vi "GUI_Beampointing2_Pico_HTU.vi"() -> ()   [LabVIEW 2020]
uses:
  Shared/GUI_Template/GUI_master/tcp_new_data_event.ctl
  Shared/GUI_Template/GUI_master/tcp new data cluster.ctl
  Ctrs/beam detection.ctl
  Ctrs/move_old.ctl
  Ctrs/stats.ctl
  General GUIs/Device GUIs/GUI_Cameras/Controls/Crosshair type def.ctl
  Ctrs/Motor Calibration.ctl
  <vilib>/Analysis/NI_AALBase.lvlib
panel:
  in  "size 2":cluster{"xhair size":dbl, "xhair size 2":dbl}={"xhair size"=20.0, "xhair size 2"=20.0} {"xhair size 2" min=0.0 max=0.0; "xhair size" min=0.0 max=0.0}
  in  "Time":timestamp[](array[timestamp])
  in  "Stats 2":T1
  in  "output cluster 2":T2
  in  "UDP error message":string
  in  "Save Stats":bool
  in  "output cluster":T6={"img to avg"=0, "beam detection para"={"Filter"=0, "Filter Para"={"X Size"=0, "Y Size"=0, "% Tolerance"=0}, "detection method"=0, "smal para"=[], "Remove small Objects"=FALSE, "Restrict to round Objects"=FALSE}, "move"={"Tolerance [%]"=0.1, "Stepsize"=0.0001, "Invert Axis"=TRUE, "Invert Direction X"=FALSE, "Invert Direction Y"=TRUE, "enable feedback"=FALSE, "Set Centriod Target"=FALSE, "my active motor"=""}, "GUIdevice 1"="", "GUIdevice 2"="", "ActiveMotor"=0, "stats path "=path ""} {"beam detection para"."smal para"."Measurement Parameter" items=["Center of Mass X", "Center of Mass Y", "First Pixel X", "First Pixel Y", "Bounding Rect Left", "Bounding Rect Top", "Bounding Rect Right", "Bounding Rect Bottom", "Max Feret Diameter Start X", "Max Feret Diameter Start Y", "Max Feret Diameter End X", "Max Feret Diameter End Y", "Max Horiz. Segment Length Left", "Max Horiz. Segment Length Right", "Max Horiz. Segment Length Row", "-", "Bounding Rect Width", "Bounding Rect Height", "Bounding Rect Diagonal", "Perimeter", "Convex Hull Perimeter", "Holes' Perimeter", "Max Feret Diameter", "Equivalent Ellipse Major Axis", "Equivalent Ellipse Minor Axis", "Equivalent Ellipse Minor Axis (Feret)", "Equivalent Rect Long Side", "Equivalent Rect Short Side", "Equivalent Rect Diagonal", "Equivalent Rect Short Side (Feret)", "Average Horiz. Segment Length", "Average Vert. Segment Length", "Hydraulic Radius", "Waddel Disk Diameter", "-", "Area", "Holes' Area", "Particle & Holes' Area", "Convex Hull Area", "Image Area", "-", "Number of Holes", "Number of Horiz. Segments", "Number of Vert. Segments", "-", "Orientation", "Max Feret Diameter Orientation", "-", "% Area/Image Area", "% Area/(Particle & Holes' Area)", "Ratio of Equivalent Ellipse Axes", "Ratio of Equivalent Rect Sides", "-", "Elongation Factor", "Compactness Factor", "Heywood Circularity Factor", "Type Factor", "-", "Sum X", "Sum Y", "Sum XX", "Sum XY", "Sum YY", "Sum XXX", "Sum XXY", "Sum XYY", "Sum YYY", "-", "Moment of Inertia XX", "Moment of Inertia XY", "Moment of Inertia YY", "Moment of Inertia XXX", "Moment of Inertia XXY", "Moment of Inertia XYY", "Moment of Inertia YYY", "Norm. Moment of Inertia XX", "Norm. Moment of Inertia XY", "Norm. Moment of Inertia YY", "Norm. Moment of Inertia XXX", "Norm. Moment of Inertia XXY", "Norm. Moment of Inertia XYY", "Norm. Moment of Inertia YYY", "Hu Moment 1", "Hu Moment 2", "Hu Moment 3", "Hu Moment 4", "Hu Moment 5", "Hu Moment 6", "Hu Moment 7"]; "beam detection para"."smal para"."Range Lower Value" format="%.2f"; "beam detection para"."smal para"."Range Upper Value" format="%.2f"; "beam detection para"."detection method" items=["clustering", "entropy", "metric", "moments", "inter-class variance"]; "beam detection para"."Filter" items=["No Filter", "Median Filter", "Low Pass Filter"]}
  in  "Trigger::1":bool
  in  "Triggerdelay::1":dbl=0.003 min=0.0 max=50000.0 format="%#_6f"
  in  "Exposure::1":dbl=0.095 min=0.0001 max=1.0 format="%#_6f"
  in  "ActiveMotorName::2":string
  in  "RelativeSettings.Axis 1.StepSize::2":dbl=50.0 caption="Axis 1 Stepsize" min=0.0 max=999999.0 format="%_4p"
  in  "RelativeSettings.Axis 3.StepSize::2":dbl=50.0 caption="Axis 2 StepSize" min=0.0 max=99999999.0 format="%_4p"
  in  "RelativeSettings.Axis 3.Position::2":dbl caption="Axis 2 Position" min=-9999990.0 max=999999.0 format="%_4p"
  in  "RelativeSettings.Axis 1.Position::2":dbl caption="Axis 1 Position" min=-999999.0 max=999999.0 format="%_4p"
  in  "RelativeMove.Axis 3.CW::2":bool caption="RelativeMove.Axis 2.CW::1"
  in  "RelativeMove.Axis 3.CCW::2":bool caption="RelativeMove.Axis. 2.CCW::1"
  in  "RelativeMove.Axis 1.CW::2":bool caption="RelativeMove.Axis 1.CW::1"
  in  "RelativeMove.Axis 1.CCW::2":bool caption="RelativeMove.Axis 1.CCW::1"
  out "Names":string[](array[string])=["PA2_Input1", "PA2_Input2", "L2_TelInpFar", "L1_TelInpNear", "L4_TREXPASS1", "L5_TREXPass2", "L6_TREXPass3", "L7_TREXPass4", "L8_M10Leak", "B1_TelInput", "B2_TelLens1"]
  in  "ActiveMotor":u16(ring)=7 items=["PA2_Input1", "PA2_Input2", "L2_TelInpFar", "L1_TelInpNear", "StretcherOut"]
  in  "Set Centriod Target":bool
  in  "size":dbl=10.299999999999997
  in  "Tab Control 2":enum32{"CCD Original ", "CCD Detected"}(tab)=enum."CCD Detected"
  out "image::1":T7(plugin-control) caption="StagingM1Far"
  out "Beam":T7(plugin-control)
  in  "Reset History":bool
  out "centriod X":dbl[](graph)=[249.59745762711864, 249.9873417721519, 249.85593220338984]
  out "centriod Y":dbl[](graph)=[256.39830508474574, 256.0126582278481, 257.0]
  out "Stats":cluster{timestamp[], dbl[]}[](graph)
  in  "Tab Control":enum32{"System", "Detection", "Feedback"}(tab)=enum."Feedback"
  in  "Save Stats":bool
  in  "update speed [ms]":i32=200
  in  "img to avg":i32=20
  in  "Save Config":bool
  in  "Load Config":bool
  in  "Cameras":u16(ring)=15 items=["10TW_Driver_Spot_Cam", "B1_TelInput", "B2_TelLens1", "B3_TelLens2", "B5_CompressorOut", "B6_SwitchYNear", "B9_OAPFront", "GIGEtest", "L1_TelInpNear", "L2_TelInpFar", "L3_TelescopeOut", "L4_TREXpass1", "L5_TREXPass2", "L6_TREXpass3", "L7_TREXPass4", "L8_M10Leak", "OAPtestCam", "PA2_Input1", "PA2_Input2", "PaperCam", "StagingAlignBeam1", "StagingAlignBeam2", "StagingCapAlignment", "StagingCapSpec", "StagingCapSpec1stOrder", "StagingChromaxGuppy", "StagingDiodeMonitor", "StagingFocusBeam1", "StagingFocusBeam2", "StagingGuppy", "StagingM1Far", "StagingM1Near", "StagingM3Far", "StagingM4", "StagingM5", "StagingMagnetCam1", "StagingMagnetCam2", "StagingMagnetCam3", "StagingManta2", "StagingModeImager2", "StagingModeTemp", "StagingOAP1Far", "StagingOAP1Near", "StagingOAP2Far", "StagingOAP2Near", "StagingPhasics", "StagingPhosphor", "StagingTapeCam", "StagingTapeMonitorCam", "StagingTopView", "TargetCam10Hz_Diode", "TargetCam1Hz_Pulsed", "TREXVarianCam0", "TREXVarianCam1", "TREXVarianCam2", "TREXVarianCam3", "TREX_CapSideView", "TREX_TA6", "TS-253a_in", "TS-CapSideview", "TS-CapSpec", "TS-ChromexCam", "TS-InputNearField", "TS-Mode1", "TS-OverlapCam", "TS-Periscope", "XUV_Cam1", "XUV_Cam2"]
  in  "calibrate":bool
  in  "stats path":path
  in  "beam detection para":T3={"Filter"=1, "Filter Para"={"X Size"=5, "Y Size"=5, "% Tolerance"=1}, "detection method"=4, "smal para"=[{"Measurement Parameter"=35, "Range Lower Value"=150.0, "Range Upper Value"=300.0, "Range"=FALSE, "Measurement Type"=FALSE}], "Remove small Objects"=TRUE, "Restrict to round Objects"=FALSE} {"smal para"."Measurement Parameter" items=["Center of Mass X", "Center of Mass Y", "First Pixel X", "First Pixel Y", "Bounding Rect Left", "Bounding Rect Top", "Bounding Rect Right", "Bounding Rect Bottom", "Max Feret Diameter Start X", "Max Feret Diameter Start Y", "Max Feret Diameter End X", "Max Feret Diameter End Y", "Max Horiz. Segment Length Left", "Max Horiz. Segment Length Right", "Max Horiz. Segment Length Row", "-", "Bounding Rect Width", "Bounding Rect Height", "Bounding Rect Diagonal", "Perimeter", "Convex Hull Perimeter", "Holes' Perimeter", "Max Feret Diameter", "Equivalent Ellipse Major Axis", "Equivalent Ellipse Minor Axis", "Equivalent Ellipse Minor Axis (Feret)", "Equivalent Rect Long Side", "Equivalent Rect Short Side", "Equivalent Rect Diagonal", "Equivalent Rect Short Side (Feret)", "Average Horiz. Segment Length", "Average Vert. Segment Length", "Hydraulic Radius", "Waddel Disk Diameter", "-", "Area", "Holes' Area", "Particle & Holes' Area", "Convex Hull Area", "Image Area", "-", "Number of Holes", "Number of Horiz. Segments", "Number of Vert. Segments", "-", "Orientation", "Max Feret Diameter Orientation", "-", "% Area/Image Area", "% Area/(Particle & Holes' Area)", "Ratio of Equivalent Ellipse Axes", "Ratio of Equivalent Rect Sides", "-", "Elongation Factor", "Compactness Factor", "Heywood Circularity Factor", "Type Factor", "-", "Sum X", "Sum Y", "Sum XX", "Sum XY", "Sum YY", "Sum XXX", "Sum XXY", "Sum XYY", "Sum YYY", "-", "Moment of Inertia XX", "Moment of Inertia XY", "Moment of Inertia YY", "Moment of Inertia XXX", "Moment of Inertia XXY", "Moment of Inertia XYY", "Moment of Inertia YYY", "Norm. Moment of Inertia XX", "Norm. Moment of Inertia XY", "Norm. Moment of Inertia YY", "Norm. Moment of Inertia XXX", "Norm. Moment of Inertia XXY", "Norm. Moment of Inertia XYY", "Norm. Moment of Inertia YYY", "Hu Moment 1", "Hu Moment 2", "Hu Moment 3", "Hu Moment 4", "Hu Moment 5", "Hu Moment 6", "Hu Moment 7"]; "smal para"."Range Lower Value" format="%.2f"; "smal para"."Range Upper Value" format="%.2f"; "detection method" items=["clustering", "entropy", "metric", "moments", "inter-class variance"]; "Filter" items=["No Filter", "Median Filter", "Low Pass Filter"]}
  in  "Move Properties":T5={"Tolerance [%]"=0.1, "Stepsize"=0.0001, "Invert Axis"=TRUE, "Invert Direction X"=FALSE, "Invert Direction Y"=TRUE, "enable feedback"=FALSE, "Set Centriod Target"=FALSE, "my active motor"=""} {"Stepsize" format="%#_6p"}
  out "Y Size":dbl=20.599999999999994
  out "X Size":dbl=15.599999999999994
  out "Particle Reports (Pixels)":T8(array[cluster])=[{"Area"=236.0, "Number of Holes"=0.0, "Bounding Rect"={"Left"=243.0, "Top"=247.0, "Right"=258.0, "Bottom"=268.0}, "Center of Mass"={"X"=249.85593220338984, "Y"=257.0}, "Orientation"=87.89795034558499, "Dimensions"={"Width"=15.0, "Height"=21.0}}] {"Orientation" format="%.2f"; "Dimensions"."Height" format="%.2f"; "Dimensions"."Width" format="%.2f"; "Center of Mass"."Y" format="%.2f"; "Center of Mass"."X" format="%.2f"; "Bounding Rect"."Bottom" format="%.2f"; "Bounding Rect"."Right" format="%.2f"; "Bounding Rect"."Top" format="%.2f"; "Bounding Rect"."Left" format="%.2f"; "Number of Holes" format="%.2f"; "Area" format="%.2f"}
  out "move required":bool=TRUE
  out "moving":bool
  out "Best Rectangle":T9(array[cluster])=[{"Left"=243.0, "Top"=247.0, "Right"=259.0, "Bottom"=267.0}, {"Left"=242.0, "Top"=246.0, "Right"=257.0, "Bottom"=267.0}, {"Left"=242.0, "Top"=246.0, "Right"=258.0, "Bottom"=267.0}, {"Left"=243.0, "Top"=247.0, "Right"=258.0, "Bottom"=268.0}, {"Left"=242.0, "Top"=247.0, "Right"=258.0, "Bottom"=267.0}]
  out "XY Graph":cluster{timestamp[], dbl[]}[](graph)
  out "Y offset":dbl=-1.5635377104373447
  out "X offset":dbl=10.405838585398385
  in  "Target.X::1":dbl=260.0 min=0.0 max=2000.0 format="%#_6f"
  in  "Target.Y::1":dbl=255.0 min=0.0 max=2000.0 format="%#_6f"
  out "mean Y":dbl=256.56353771043734 format="%0.2f"
  out "mean X":dbl=249.59416141460161 format="%0.2f"
  out "beam detected":bool=TRUE
  in  "GUIdevice 2":string="U_148_PicoServer"
  out "error out":errorcluster
  in  "insert tag":bool=TRUE
  in  "stop":bool=TRUE
  in  "GUIdevice 1":string="UC_Amp2_IR_input"
  out "tcp data event":T10
  out "error IO 2":errorcluster
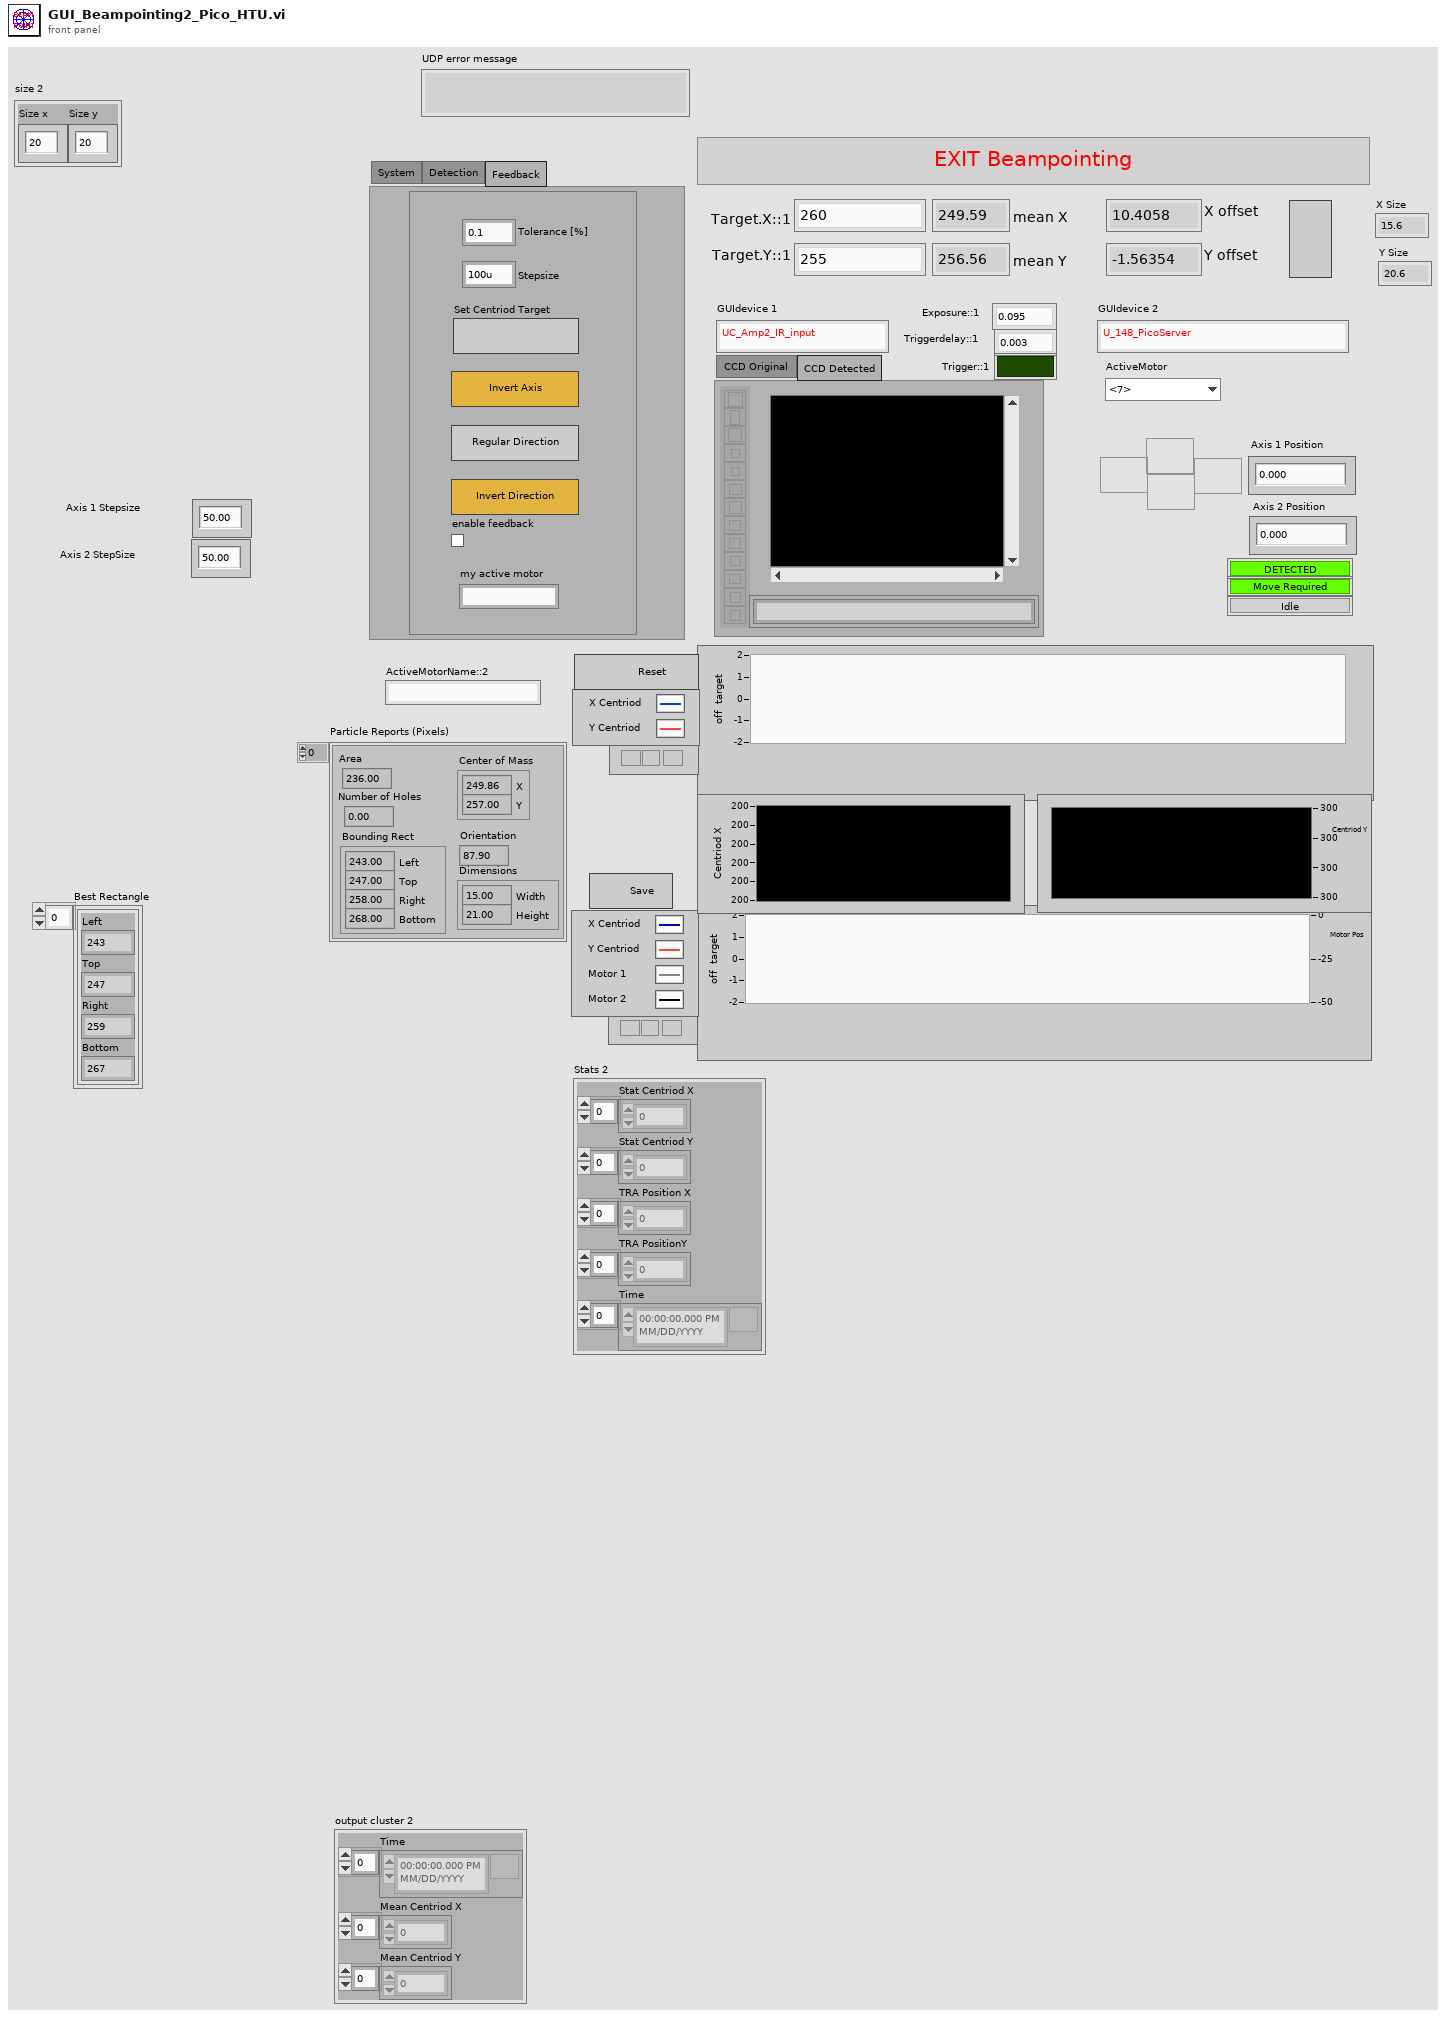
[diagram p1: front panel]
types:
  T1 = typedef "stats.ctl" = cluster{"Stat Centriod X":dbl[], "Stat Centriod Y":dbl[], "TRA Position X":dbl[], "TRA PositionY":dbl[], "Time":timestamp[]}
  T2 = cluster{"Time":timestamp[], "Mean Centriod X":dbl[], "Mean Centriod Y":dbl[]}
  T3 = typedef "beam detection.ctl" = cluster{"Filter":u16, "Filter Para":cluster{"X Size":i32, "Y Size":i32, "% Tolerance":i32}, "detection method":i32, "smal para":cluster{"Measurement Parameter":T4, "Range Lower Value":dbl, "Range Upper Value":dbl, "Range":bool, "Measurement Type":bool}[], "Remove small Objects":bool, "Restrict to round Objects":bool}
  T4 = typedef "Particle Parameters" = i32
  T5 = typedef "move_old.ctl" = cluster{"Tolerance [%]":dbl, "Stepsize":dbl, "Invert Axis":bool, "Invert Direction X":bool, "Invert Direction Y":bool, "enable feedback":bool, "Set Centriod Target":bool, "my active motor":string}
  T6 = cluster{"img to avg":i32, "beam detection para":T3, "move":T5, "GUIdevice 1":string, "GUIdevice 2":string, "ActiveMotor":u16, "stats path ":path}
  T7 = typedef "IMAQ Image.ctl" = refnum<image>
  T8 = cluster{"Area":dbl, "Number of Holes":dbl, "Bounding Rect":cluster{"Left":dbl, "Top":dbl, "Right":dbl, "Bottom":dbl}, "Center of Mass":cluster{"X":dbl, "Y":dbl}, "Orientation":dbl, "Dimensions":cluster{"Width":dbl, "Height":dbl}}[]
  T9 = cluster{"Left":dbl, "Top":dbl, "Right":dbl, "Bottom":dbl}[]
  T10 = typedef "tcp_new_data_event.ctl" = refnum<user-event>
  T11 = typedef "tcp new data cluster.ctl" = cluster{"EventEnum":enum16{"new data", "connection status update"}, "Device name":string}
  T12 = typedef "Image Type" = u32
  T13 = cluster{"RelativeMove.Axis 1.CW::2":refnum<vi>, "RelativeMove.Axis 1.CCW::2":refnum<vi>, "RelativeMove.Axis 3.CW::2":refnum<vi>, "RelativeMove.Axis 3.CCW::2":refnum<vi>}
  T14 = typedef "Crosshair type def.ctl" = cluster{"Draw":bool, "Target":cluster{"x":dbl, "y":dbl}, "Size":cluster{"x":dbl, "y":dbl}, "Angle":dbl, "Color":u32, "Thickness":u8, "CrosshairLabel":string}
  T15 = cluster{"Left":i32, "Top":i32, "Right":i32, "Bottom":i32}
  T16 = enum32{"invalid app kind", "Development System", "Run Time System", "Student Edition", "Embedded LabVIEW", "Evaluation", "Custom"}
  T17 = enum32{"Invalid", "Standard", "Closed", "Hidden", "Minimized", "Maximized"}
  T18 = enum16{"open", "replace", "create", "open or create", "replace or create", "replace or create with confirmation"}
  T19 = typedef "Motor Calibration.ctl" = cluster{"Slope Axis 1":dbl, "Axis Inverted":bool, "Slope Axis 2":dbl, "Axis 1 revered":bool, "Axis 2 revered":bool}
  T20 = cluster{"Core":cluster{"Current VI Reference":refnum<vi>, "Close Panel on Exit?":bool}, "beam detection para":T3, "Centriod X":dbl[], "Centriod Y":dbl[], "Best Rectangle":cluster{"Left":dbl, "Top":dbl, "Right":dbl, "Bottom":dbl}[], "PArticle Report":cluster{"Area":dbl, "Number of Holes":dbl, "Bounding Rect":cluster{"Left":dbl, "Top":dbl, "Right":dbl, "Bottom":dbl}, "Center of Mass":cluster{"X":dbl, "Y":dbl}, "Orientation":dbl, "Dimensions":cluster{"Width":dbl, "Height":dbl}}[], "Mean Centriod X":dbl[], "Mean Centriod Y":dbl[], "Time":timestamp[], "beam detected":bool, "offsets":cluster{"X offset":dbl, "Y offset":dbl}, "move":T5, "moving":bool, "Stats":T1, "set centriod target":bool, "Motor Calibration":T19}
  T21 = cluster{"Left":dbl, "Top":dbl, "Right":dbl, "Bottom":dbl}
  T22 = cluster{"Current VI Reference":refnum<vi>, "Close Panel on Exit?":bool}
  T23 = cluster{"Time":timestamp[], "Stat Centriod X":dbl[]}
  T24 = cluster{"Time":timestamp[], "Stat Centriod Y":dbl[]}
  T25 = cluster{"Time":timestamp[], "TRA Position X":dbl[]}
  T26 = cluster{"Time":timestamp[], "TRA PositionY":dbl[]}
  T27 = cluster{"Time":timestamp[], "TRA PositionY":dbl[]}[]
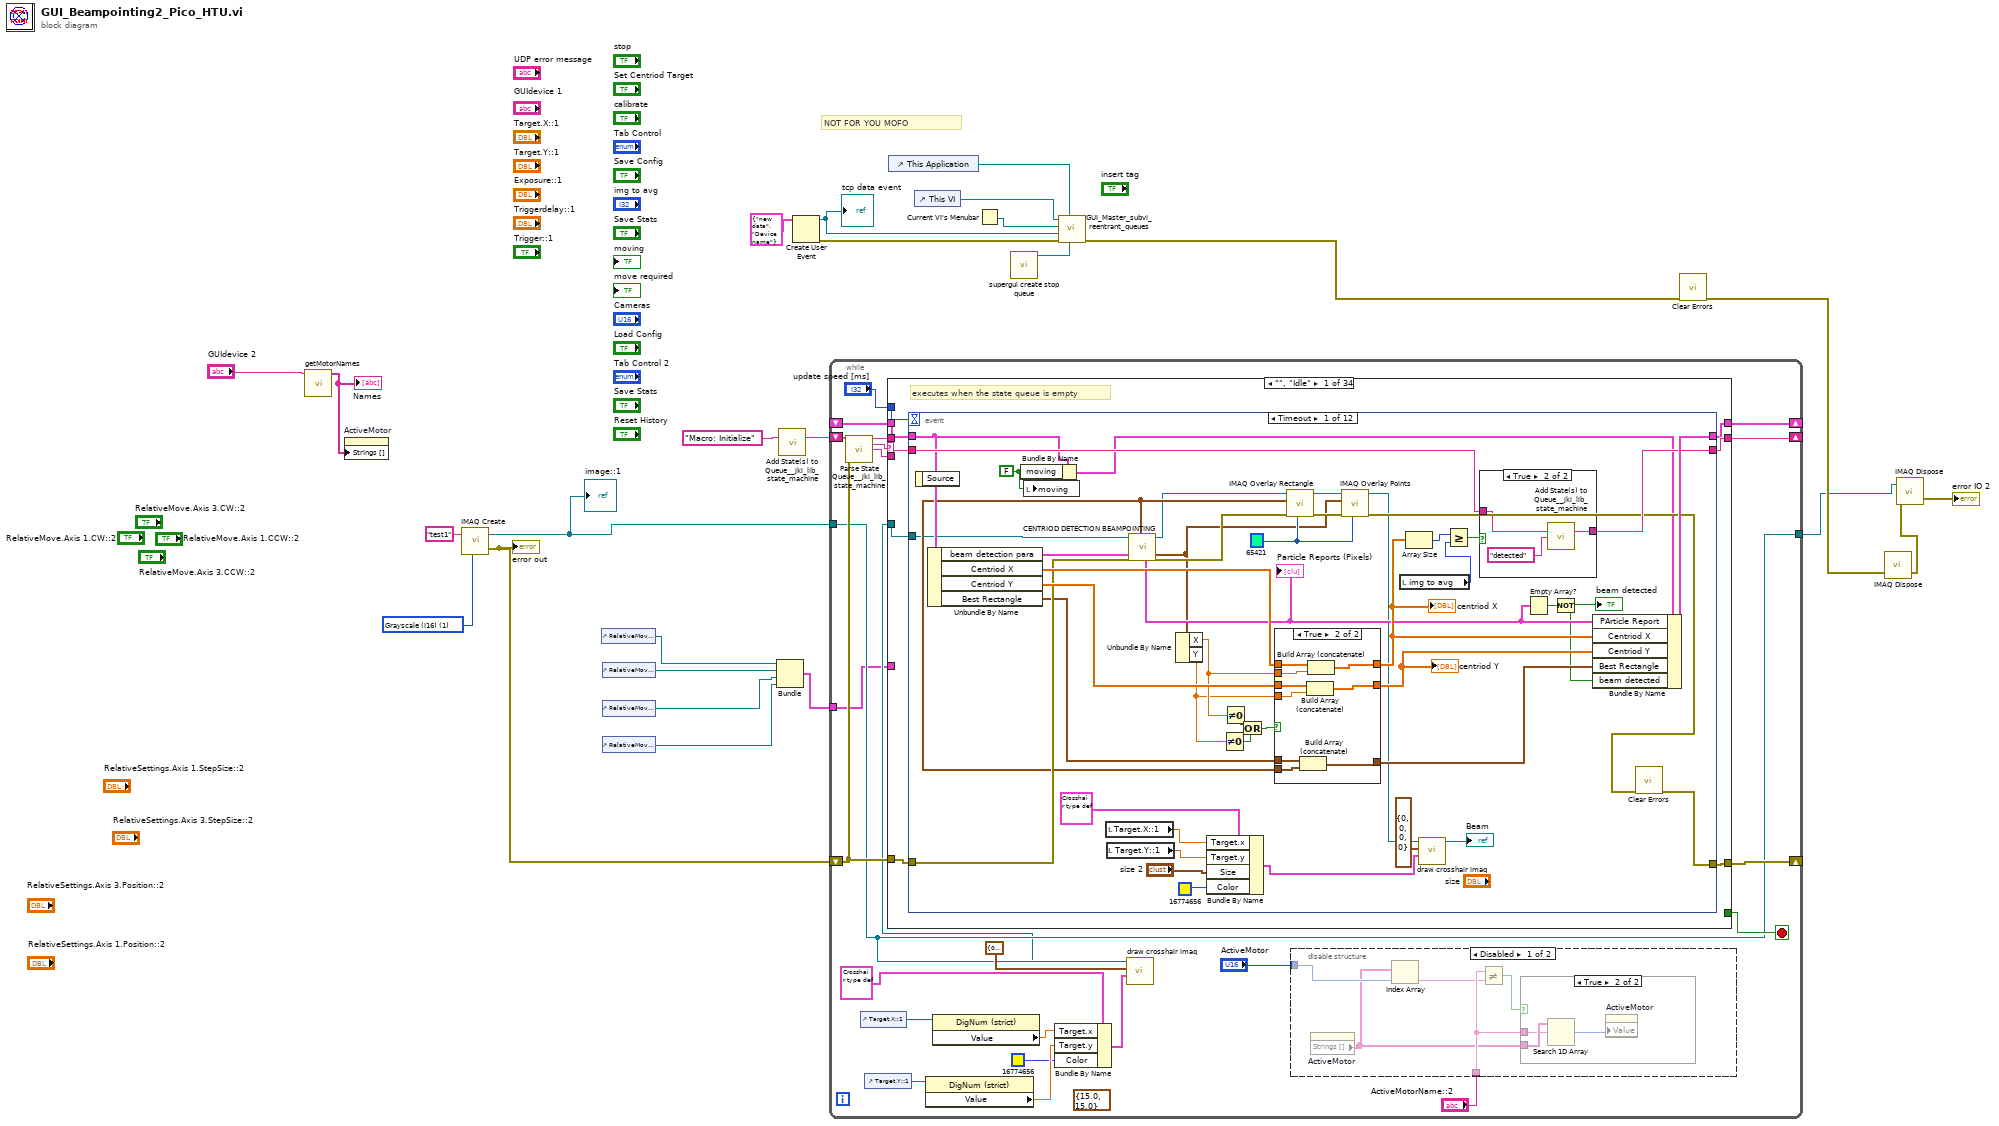
[diagram p0: block diagram]
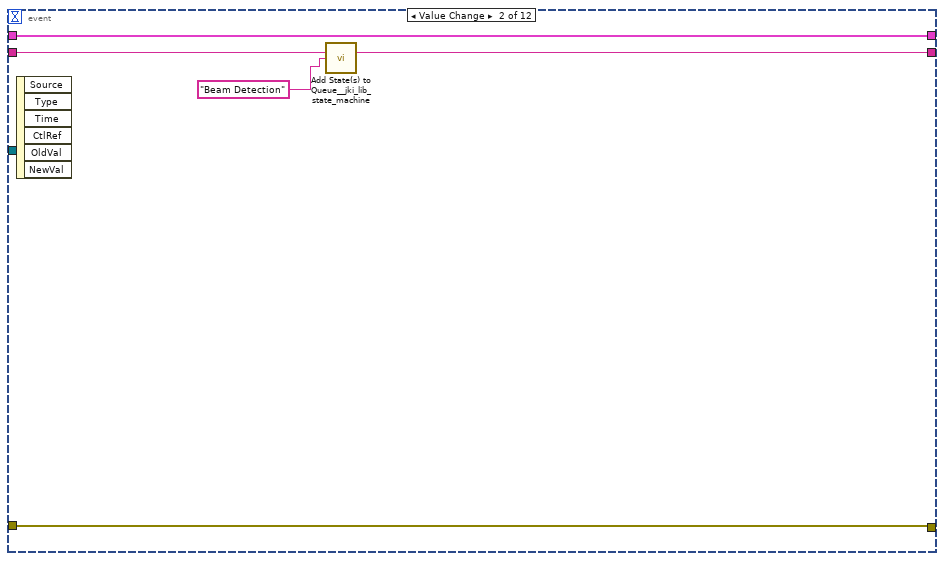
[diagram p6: hidden frame]
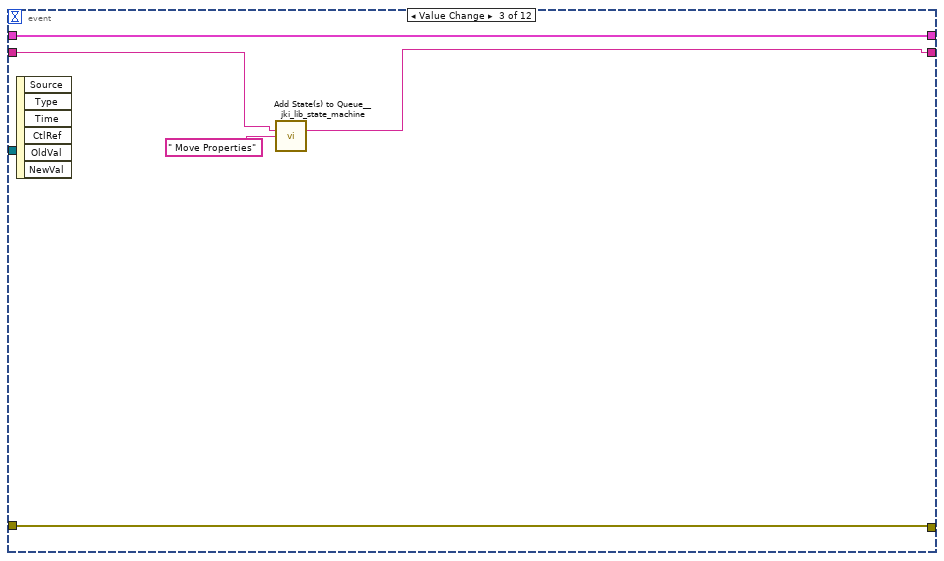
[diagram p7: hidden frame]
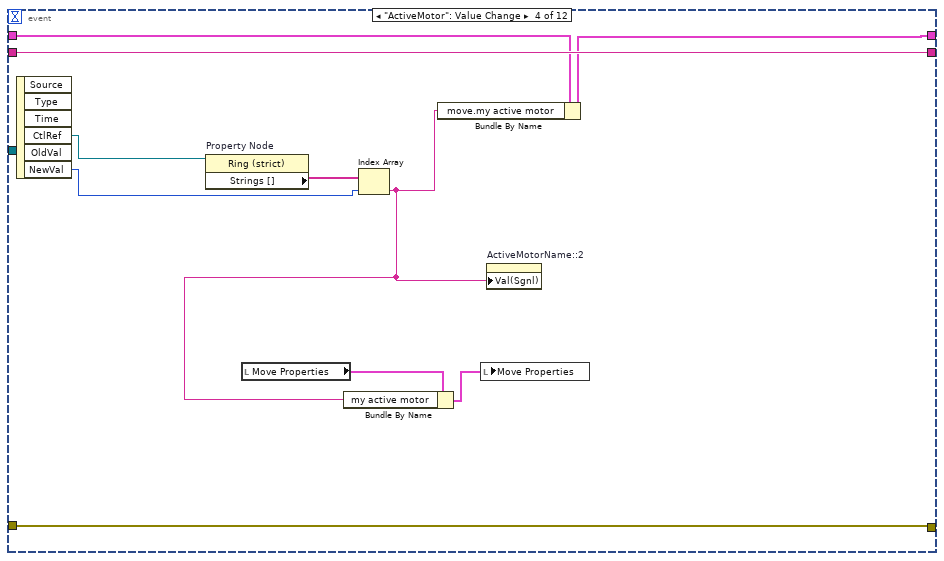
[diagram p8: hidden frame]
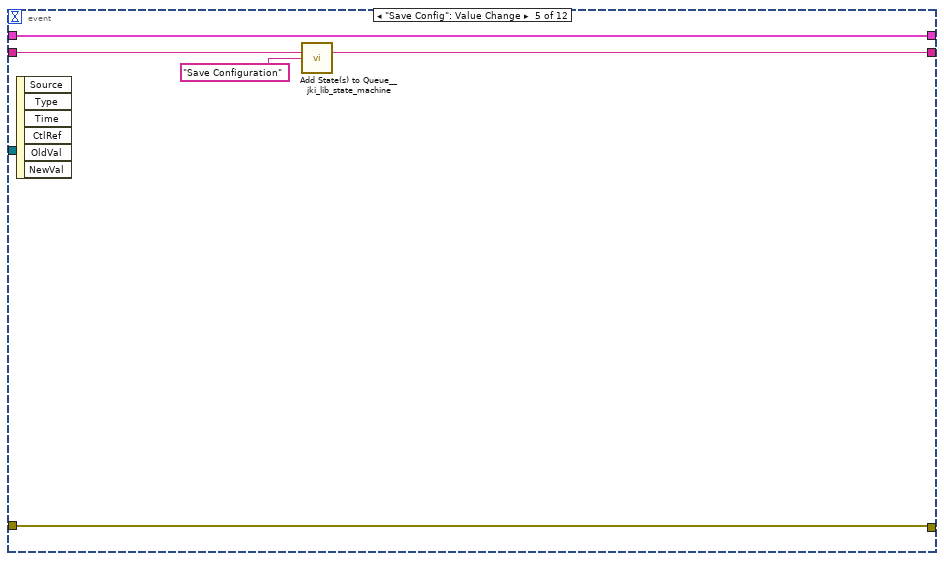
[diagram p9: hidden frame]
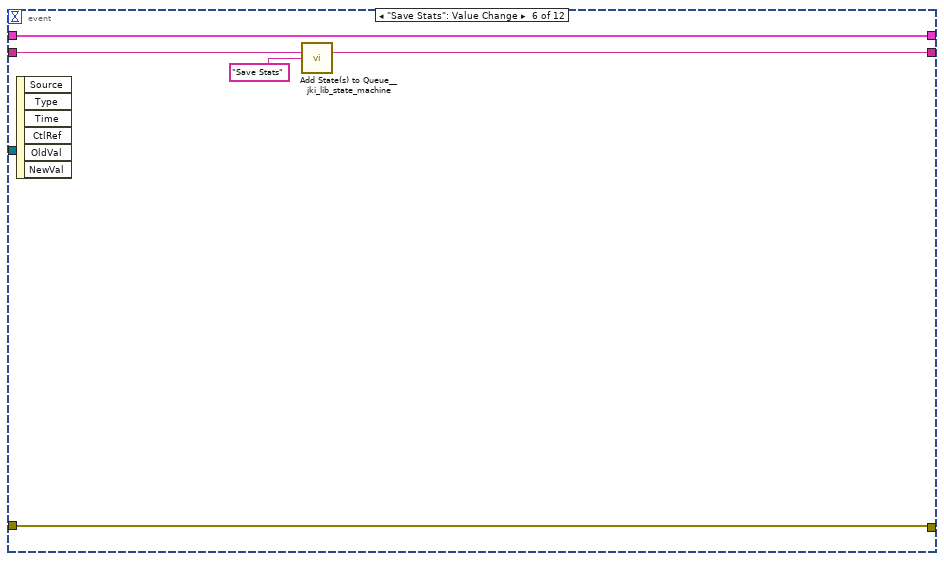
[diagram p10: hidden frame]
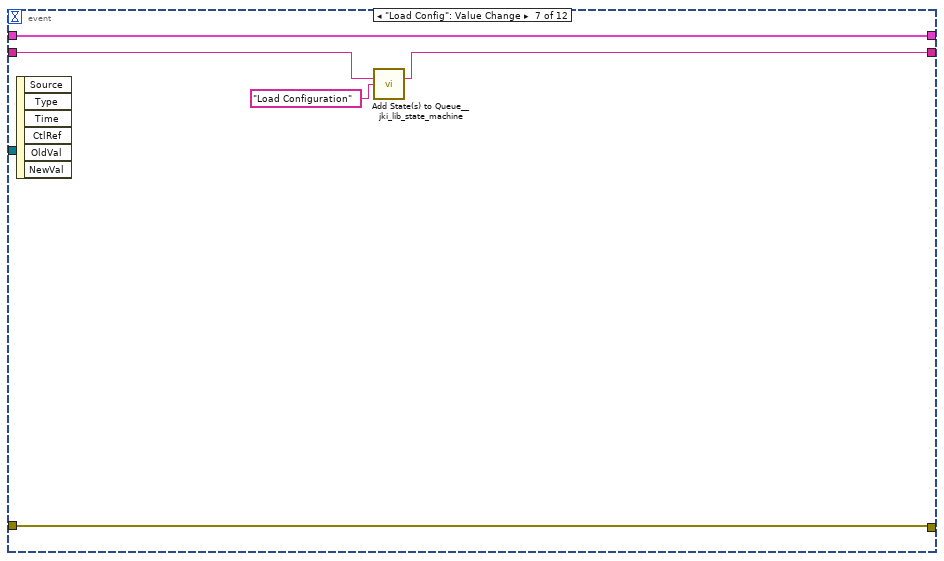
[diagram p11: hidden frame]
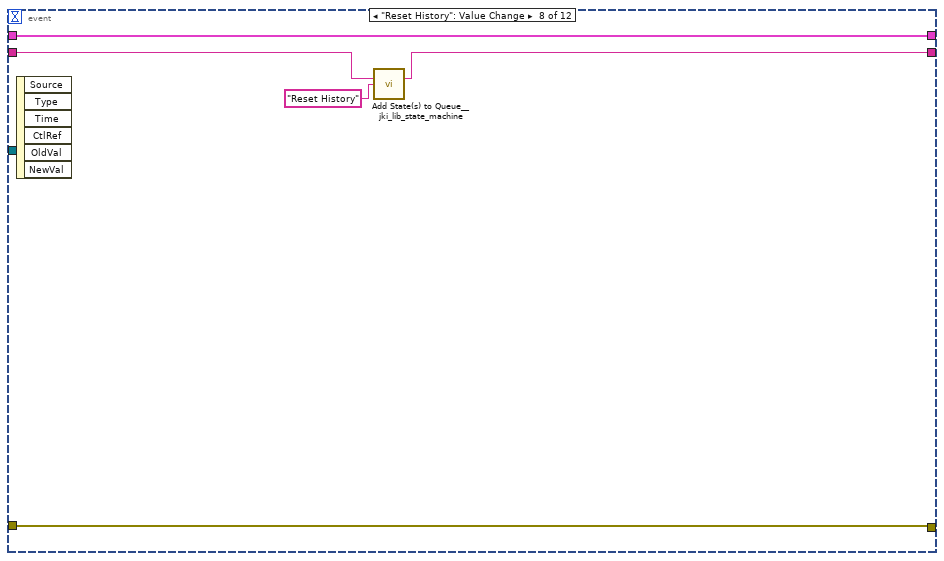
[diagram p12: hidden frame]
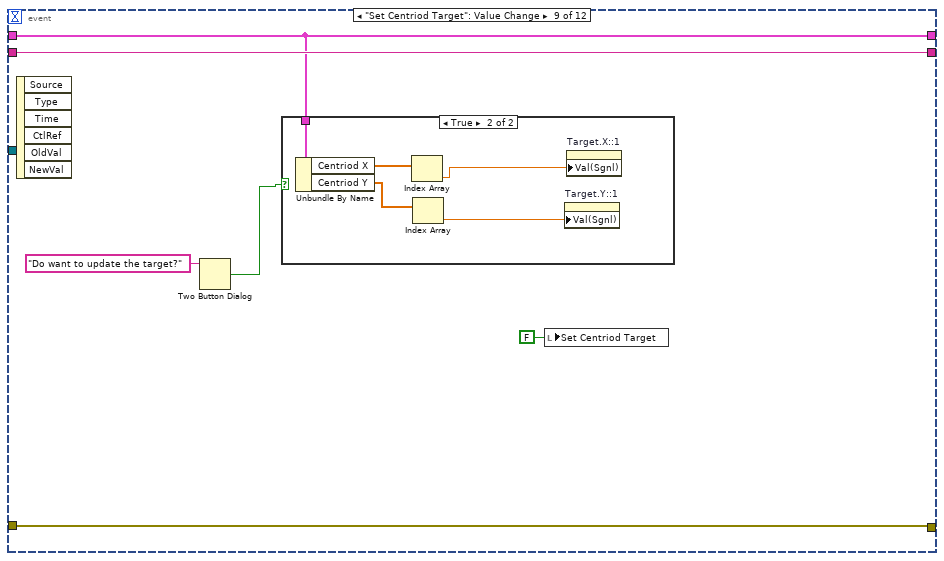
[diagram p13: hidden frame]
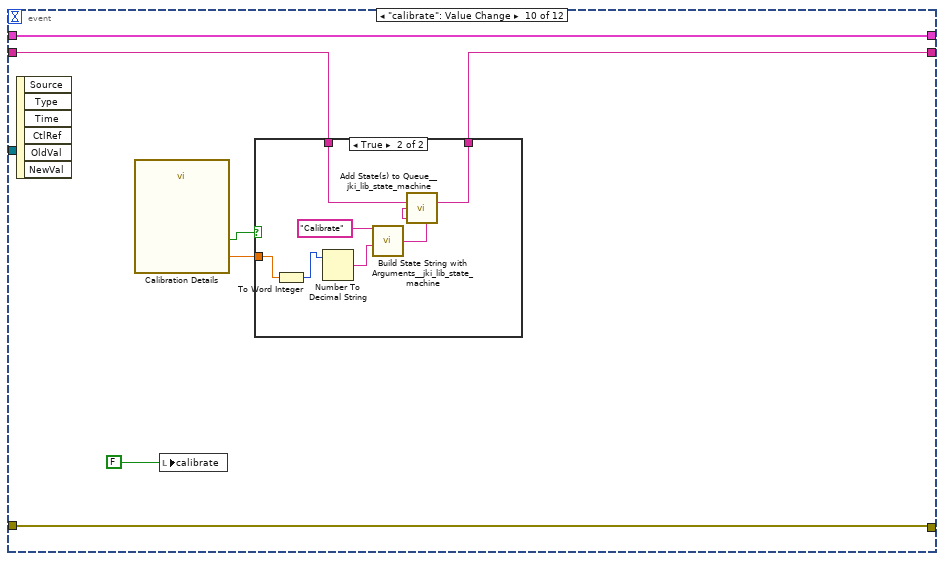
[diagram p15: hidden frame]
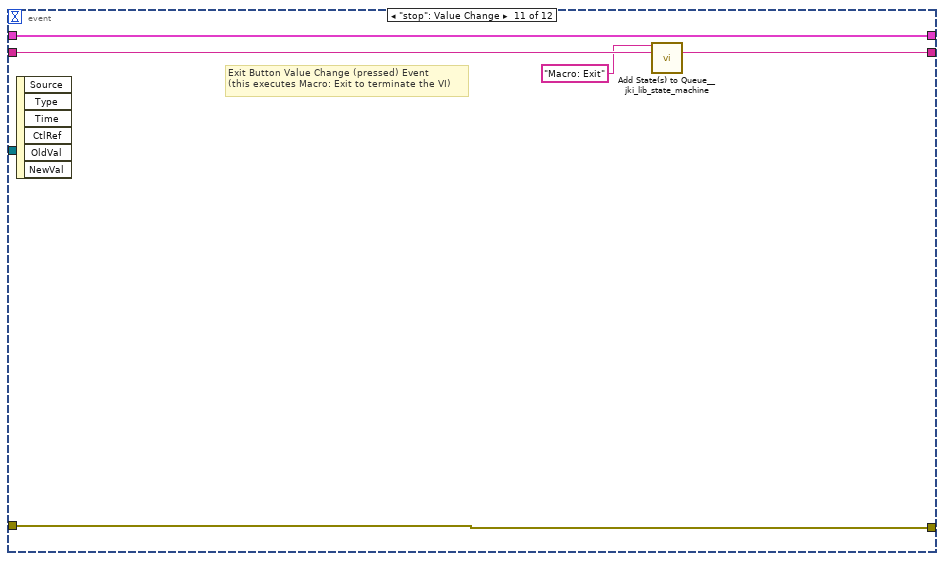
[diagram p17: hidden frame]
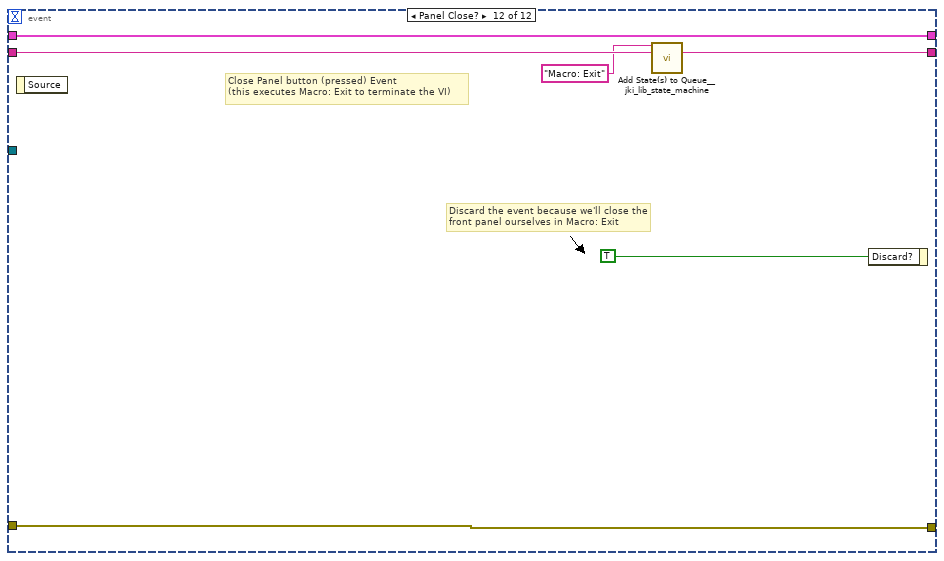
[diagram p18: hidden frame]
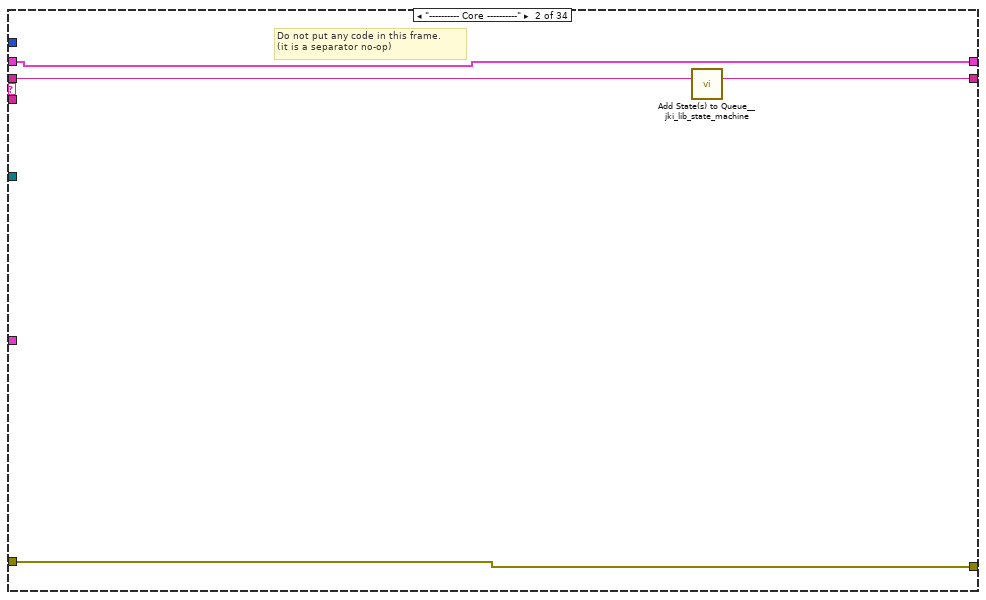
[diagram p19: hidden frame]
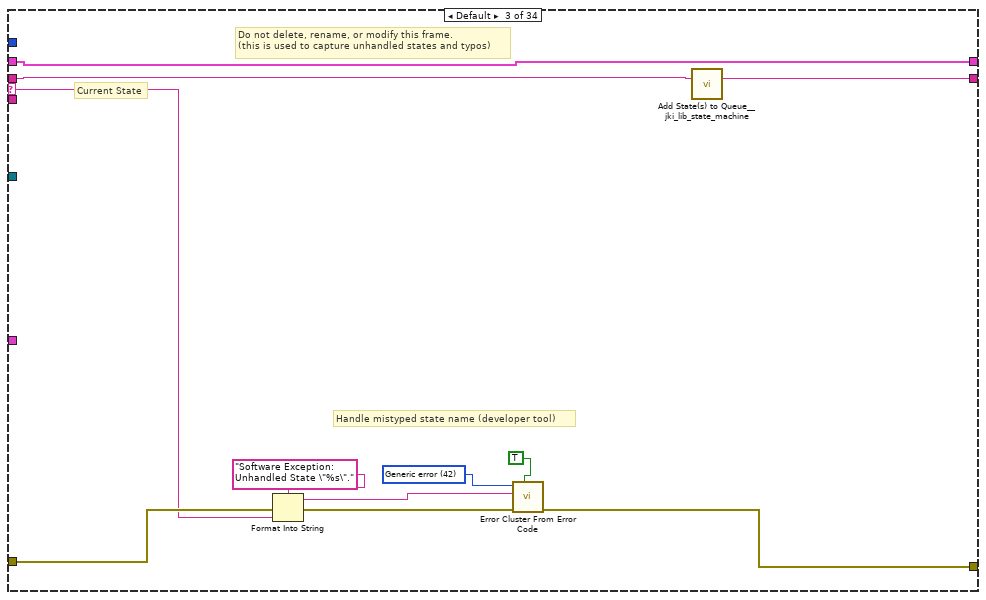
[diagram p20: hidden frame]
diagram:
  w24 = T12 1 items=["Grayscale (U8)", "Grayscale (I16)", "Grayscale (SGL)", "Complex (CSG)", "RGB (U32)", "HSL (U32)", "RGB (U64)", "Grayscale (U16)"] ("Image Type")
  # "NOT FOR YOU MOFO"
  n1 = call "getMotorNames.vi"("DeviceName"="GUIdevice 2") -> ("elements"=w7:string[])  [unwired: 10 in]
  "Names" <- w7
  n2 = property on="ActiveMotor" class="Ring (strict)"("Strings []"=w7) -> ()  [unwired: 2 in, 2 out]
  n3 = call "IMAQ Create"("Image Name"="test1", "Image Type"=w24) -> ("New Image"=w9:T7, "error out"=w17:errorcluster)  [unwired: 3 in]
  "error out" <- w17
  "image::1" <- w9
  n4 = control-ref of="RelativeMove.Axis 1.CW::2"() -> (w6:refnum<vi>)
  n5 = control-ref of="RelativeMove.Axis 1.CCW::2"() -> (w5:refnum<vi>)
  n6 = control-ref of="RelativeMove.Axis 3.CW::2"() -> (w4:refnum<vi>)
  n7 = control-ref of="RelativeMove.Axis 3.CCW::2"() -> (w3:refnum<vi>)
  n8 = Bundle("RelativeMove.Axis 1.CW::2"=w6, "RelativeMove.Axis 1.CCW::2"=w5, "RelativeMove.Axis 3.CW::2"=w4, "RelativeMove.Axis 3.CCW::2"=w3) -> (w2:T13)  [unwired: 1 in]
  n9 = call <vilib>:"Add State(s) to Queue__jki_lib_state_machine.vi"("State(s) in (\"\")"="Macro: Initialize") -> ("States Out"=w19:string)  [unwired: 14 in]
  n10 = Create User Event(user event datatype=T11 {"EventEnum"=enum."new data", "Device name"="Device name"} ("New Event")) -> (user event=w10:refnum<user-event>, error out=w12:errorcluster)  [unwired: 1 in]
  "tcp data event" <- w10
  n11 = while "JKI - String-Based Queued State Machine (Basic) v1.0" {
    shift-right: [w43] -> _
    shift-left: _ -> [w42]
    shift-right: [w45] -> _
    shift-left: w17 -> [w40]
    shift-right: [w44] -> _
    shift-left: w19 -> [w46]
    tunnel: w9 -> [w35]
    tunnel: [w35] -> w16
    tunnel: w2 -> [w33]
    stop <- w39 stop-if-true
    (unwired) cluster{"xhair size":dbl, "xhair size 2":dbl} {"xhair size"=15.0, "xhair size 2"=15.0} ("size")
    n12 = call <vilib>:"Parse State Queue__jki_lib_state_machine.vi"("State Queue"=w46, "Error In (no error)"=w40) -> ("Remaining States"=w48:string, "Current State"=w49:string, "Arguments"=w47:string)  [unwired: 11 in]
    n13 = control-ref of="Target.X::1"() -> (w37:refnum<vi>)
    n14 = control-ref of="Target.Y::1"() -> (w38:refnum<vi>)
    n15 = property class="DigNum (strict)"(reference=w38) -> ("Value"=w28:dbl)  [unwired: 1 in, 2 out]
    n16 = property class="DigNum (strict)"(reference=w37) -> ("Value"=w29:dbl)  [unwired: 1 in, 2 out]
    n17 = Bundle By Name(cluster=T14 {"Draw"=TRUE, "Target"={"x"=25.0, "y"=25.0}, "Size"={"x"=25.0, "y"=25.0}, "Angle"=0.0, "Color"=8322834, "Thickness"=1, "CrosshairLabel"=""} ("Crosshair"), "Target.x"=w29, "Target.y"=w28, "Color"=u32 16774656) -> (w27:T14)
    n18 = call "draw crosshair imaq.vi"("Crosshair"=w27, "Bounding Rectangle"=T15 {"Left"=0, "Top"=0, "Right"=0, "Bottom"=0}, "image in"=w35) -> ("image out"=w34:T7)  [unwired: 7 in, 1 out]
    n19 = case shown="\"\", \"Idle\"" w49 {
      selector: w49 -> [_ _ w207 _ _ _ _ _ _ _ _ _ _ _ _ _ _ _ _ _ _ _ _ _ _ _ _ _ _ _ _ _ _ _]
      tunnel: w48 -> [w65 w206 w211 w229 w235 w240 w244 w268 w274 w278 w282 w288 w299 w325 w330 w340 w344 w350 w357 w378 w386 w407 w443 w451 w455 w488 w498 w535 w559 w631 w691 w704 w779 w783]
      tunnel: w47 -> [_ _ _ _ _ _ _ _ _ _ _ w283 w293 _ _ _ _ _ _ _ _ _ _ _ _ _ _ _ _ _ _ w697 w774 _]
      tunnel: w42 -> [w63 w203 w209 w220 w232 w238 w241 _ w270 w275 w280 w286 w295 w322 w327 w337 w341 w346 w353 w361 w384 w405 w435 w447 w452 w471 w500 w532 w546 w618 w687 w726 w776 w780]
      tunnel: [w62 w204 w213 w226 errorcluster {"status"=FALSE, "code"=0, "source"=""} ("error out") w237 w242 w265 w271 w276 w279 w284 w296 w323 w328 w338 w342 w348 w355 w366 w382 w403 w432 w449 w453 w487 w519 w533 w557 w629 w680 w728 w775 w781] -> w45
      tunnel: w40 -> [w61 w204 w212 w226 w231 w237 w242 w265 w272 w276 w279 w285 w297 w323 w328 w338 w342 w348 w355 w367 w383 w404 w433 w449 w453 w487 w519 w533 w557 w629 w681 w728 w775 w781]
      tunnel: [w64 w205 w210 w228 w234 w239 w243 w267 w273 w277 w281 w287 w298 w324 w329 w339 w343 w349 w356 w377 w385 w406 w442 w450 w454 w456 w506 w534 w558 w630 w690 w729 w778 w782] -> w44
      tunnel: [_ _ _ _ _ TRUE _ _ _ _ _ _ _ _ _ _ _ _ _ _ _ _ _ _ _ _ _ _ _ _ _ _ _ _] -> w39
      tunnel: [w60 w203 w209 w227 w232 w238 w241 w266 w270 w275 w280 w286 w295 w322 w327 w337 w341 w345 w352 w361 w384 w405 w434 w446 w452 w470 w504 w532 w556 w628 w688 w716 w776 w780] -> w43
      tunnel: "update speed [ms]" -> [w59 _ _ _ _ _ _ _ _ _ _ _ _ _ _ _ _ _ _ _ _ _ _ _ _ _ _ _ _ _ _ _ _ _]
      tunnel: w34 -> [w58 _ _ _ _ _ _ _ _ _ _ _ _ _ _ _ _ _ _ _ _ _ _ _ _ _ _ _ _ _ _ _ w773 _]
      tunnel: w33 -> [_ _ _ _ _ _ _ _ _ _ _ _ _ _ _ _ _ _ _ _ _ _ _ _ _ _ _ _ w551 w623 _ _ w777 _]
      frame "", "Idle" {
        # "executes when the state queue is empty"
        n20 = event shown="[0] Timeout" {
          selector: _ -> [_ _ _ _ _ _ _ _ _ _ _ _]
          dyn-events: _ -> [_ _ _ _ _ _ _ _ _ _ _ _]
          timeout: w59 -> [_ _ _ _ _ _ _ _ _ _ _ _]
          tunnel: w65 -> [w91 w129 w134 w141 w149 w154 w158 w163 w170 w180 w196 w202]
          tunnel: [w90 w128 w132 w141 w147 w152 w157 w162 w170 w179 w195 w201] -> w64
          tunnel: w63 -> [w81 w130 w135 w140 w150 w155 w160 w165 w169 w182 w193 w199]
          tunnel: [w87 w127 w131 w142 w146 w151 w159 w164 w171 w183 w194 w200] -> w62
          tunnel: w61 -> [w105 w127 w131 w142 w146 w151 w159 w164 w171 w183 w194 w200]
          tunnel: [w108 w130 w135 w139 w150 w155 w160 w165 w169 w182 w193 w199] -> w60
          tunnel: w58 -> [w67 _ _ _ _ _ _ _ _ _ _ _]
          event Timeout {
            w79 = FALSE ("moving")
            w97 = u32 65421 ("Color")
            n21 = event-data() -> ()  [unwired: 1 in, 1 out]
            n22 = Unbundle By Name(w81) -> ("beam detection para"=w109:T3, "Centriod X"=w107:dbl[], "Centriod Y"=w106:dbl[], "Best Rectangle"=w99:T9)
            n23 = Bundle By Name(cluster=w81, "moving"=w79) -> (w80:T20)
            n24 = local write "moving"(w79) -> ()
            n25 = local read "Target.X::1"() -> (w73:dbl)
            n26 = local read "Target.Y::1"() -> (w72:dbl)
            n27 = call "CENTRIOD DETECTION BEAMPOINTING.vi"("Refnum in"=w67, "beam detection para"=w109, "error in (no error)"=w105) -> ("Bounding Rect"=w75:T21, "Particle Reports (Pixels)"=w84:T8, "Refnum out"=w66:T7, "Centriod"=w76:cluster{"X":dbl, "Y":dbl}, "error out"=w89:errorcluster)  [unwired: 10 in, 2 out]
            "Particle Reports (Pixels)" <- w84
            n28 = Unbundle By Name(w76) -> ("X"=w102:dbl, "Y"=w101:dbl)
            n29 = Bundle By Name(cluster=T14 {"Draw"=TRUE, "Target"={"x"=25.0, "y"=25.0}, "Size"={"x"=25.0, "y"=25.0}, "Angle"=0.0, "Color"=8322834, "Thickness"=1, "CrosshairLabel"=""} ("Crosshair"), "Target.x"=w73, "Target.y"=w72, "Size"="size 2", "Color"=u32 16774656) -> (w70:T14)
            n30 = Not Equal To 0?(x=w101) -> (x != 0?=w104:bool)
            n31 = Not Equal To 0?(x=w102) -> (x != 0?=w103:bool)
            n32 = Or(x=w103, y=w104) -> (x .or. y?=w100:bool)
            n33 = case shown="True" w100 {
              tunnel: w107 -> [w116 w125]
              tunnel: w106 -> [w115 w124]
              tunnel: [w116 w123] -> w93
              tunnel: [w115 w122] -> w94
              tunnel: w102 -> [_ w121]
              tunnel: w101 -> [_ w120]
              tunnel: w99 -> [w114 w119]
              tunnel: w75 -> [_ w118]
              tunnel: [w114 w117] -> w98
              frame False {
              }
              frame True {
                n34 = Build Array (concatenate)(w119, w118) -> (w117:T9)
                n35 = Build Array (concatenate)(w124, w120) -> (w122:dbl[])
                n36 = Build Array (concatenate)(w125, w121) -> (w123:dbl[])
              }
            }
            "centriod X" <- w93
            "centriod Y" <- w94
            n37 = call "IMAQ Overlay Rectangle"("Color"=w97, "error in (no error)"=w89, "Rectangle"=w75, "Image"=w66) -> ("error out"=w95:errorcluster, "Image Out"=w96:T7)  [unwired: 6 in]
            n38 = call "IMAQ Overlay Points"("Color"=w97, "error in (no error)"=w95, "Point"=w76, "Image"=w96) -> ("error out"=w88:errorcluster, "Image Out"=w68:T7)  [unwired: 6 in]
            n39 = local read "img to avg"() -> (w85:i32)
            n40 = Array Size(array=w93) -> (size(s)=w86:i32)
            n41 = call "draw crosshair imaq.vi"("Crosshair"=w70, "Bounding Rectangle"=T15 {"Left"=0, "Top"=0, "Right"=0, "Bottom"=0}, "image in"=w68) -> ("image out"=→"Beam":T7)  [unwired: 7 in, 1 out]
            n42 = Greater Or Equal?(x=w86, y=w85) -> (x >= y?=w92:bool)
            n43 = case shown="True" w92 {
              tunnel: w91 -> [w110 w113]
              tunnel: [w110 w112] -> w90
              frame False {
              }
              frame True {
                n44 = call <vilib>:"Add State(s) to Queue__jki_lib_state_machine.vi"("State(s) in (\"\")"=w113, "State(s) at Back (\"\")"="detected" ("State(s) in Front (\"\")")) -> ("States Out"=w112:string)  [unwired: 13 in]
              }
            }
            n45 = Empty Array?(array=w84) -> (empty?=w83:bool)
            n46 = Not(x=w83) -> (.not. x?=w82:bool)
            "beam detected" <- w82
            n47 = Bundle By Name(cluster=w80, "PArticle Report"=w84, "Centriod X"=w93, "Centriod Y"=w94, "Best Rectangle"=w98, "beam detected"=w82) -> (w108:T20)
            n48 = call <vilib>:"Clear Errors.vi"("error in (no error)"=w88) -> ("error out"=w87:errorcluster)  [unwired: 5 in, 1 out]
          }
          event Value Change {
            n49 = event-data() -> ()  [unwired: 1 in, 6 out]
            n50 = call <vilib>:"Add State(s) to Queue__jki_lib_state_machine.vi"("State(s) in (\"\")"=w129, "State(s) at Back (\"\")"="Beam Detection" ("State(s) at Back (\"\")")) -> ("States Out"=w128:string)  [unwired: 13 in]
          }
          event Value Change {
            n51 = event-data() -> ()  [unwired: 1 in, 6 out]
            n52 = call <vilib>:"Add State(s) to Queue__jki_lib_state_machine.vi"("State(s) in (\"\")"=w134, "State(s) at Back (\"\")"=" Move Properties" ("State(s) at Back (\"\")")) -> ("States Out"=w132:string)  [unwired: 13 in]
          }
          event "ActiveMotor": Value Change {
            n53 = event-data() -> ("CtlRef"=w144:refnum<vi>, "NewVal"=w143:u16)  [unwired: 1 in, 4 out]
            n54 = property on="Property Node" class="Ring (strict)"(reference=w144) -> ("Strings []"=w145:string[])  [unwired: 1 in, 2 out]
            n55 = local read "Move Properties"() -> (w138:T5)
            n56 = Index Array(array=w145, index=w143) -> (element=w137:string)
            n57 = Bundle By Name(cluster=w138, "my active motor"=w137) -> (w136:T5)
            n58 = Bundle By Name(cluster=w140, "move.my active motor"=w137) -> (w139:T20)
            n59 = local write "Move Properties"(w136) -> ()
            n60 = property on="ActiveMotorName::2" class="Str"("Val(Sgnl)"=w137) -> ()  [unwired: 2 in, 2 out]
          }
          event "Save Config": Value Change {
            n61 = event-data() -> ()  [unwired: 1 in, 6 out]
            n62 = call <vilib>:"Add State(s) to Queue__jki_lib_state_machine.vi"("State(s) in (\"\")"=w149, "State(s) at Back (\"\")"="Save Configuration" ("State(s) in Front (\"\")")) -> ("States Out"=w147:string)  [unwired: 13 in]
          }
          event "Save Stats": Value Change {
            n63 = event-data() -> ()  [unwired: 1 in, 6 out]
            n64 = call <vilib>:"Add State(s) to Queue__jki_lib_state_machine.vi"("State(s) in (\"\")"=w154, "State(s) at Back (\"\")"="Save Stats" ("State(s) in Front (\"\")")) -> ("States Out"=w152:string)  [unwired: 13 in]
          }
          event "Load Config": Value Change {
            n65 = event-data() -> ()  [unwired: 1 in, 6 out]
            n66 = call <vilib>:"Add State(s) to Queue__jki_lib_state_machine.vi"("State(s) in (\"\")"=w158, "State(s) at Back (\"\")"="Load Configuration" ("State(s) in Front (\"\")")) -> ("States Out"=w157:string)  [unwired: 13 in]
          }
          event "Reset History": Value Change {
            n67 = event-data() -> ()  [unwired: 1 in, 6 out]
            n68 = call <vilib>:"Add State(s) to Queue__jki_lib_state_machine.vi"("State(s) in (\"\")"=w163, "State(s) at Back (\"\")"="Reset History" ("State(s) in Front (\"\")")) -> ("States Out"=w162:string)  [unwired: 13 in]
          }
          event "Set Centriod Target": Value Change {
            n69 = event-data() -> ()  [unwired: 1 in, 6 out]
            n70 = Two Button Dialog(message="Do want to update the target?") -> (T button?=w166:bool)  [unwired: 2 in]
            n71 = case shown="True" w166 {
              tunnel: w169 -> [_ w176]
              frame False {
              }
              frame True {
                n72 = Unbundle By Name(w176) -> ("Centriod X"=w175:dbl[], "Centriod Y"=w173:dbl[])
                n73 = Index Array(array=w175) -> (element=w174:dbl)  [unwired: 1 in]
                n74 = Index Array(array=w173) -> (element=w172:dbl)  [unwired: 1 in]
                n75 = property on="Target.Y::1" class="DigNum (strict)"("Val(Sgnl)"=w172) -> ()  [unwired: 2 in, 2 out]
                n76 = property on="Target.X::1" class="DigNum (strict)"("Val(Sgnl)"=w174) -> ()  [unwired: 2 in, 2 out]
              }
            }
            n77 = local write "Set Centriod Target"(FALSE ("Set Centriod Target")) -> ()
          }
          event "calibrate": Value Change {
            n78 = event-data() -> ()  [unwired: 1 in, 6 out]
            n79 = call "Calibration Details"() -> ("Number of Steps"=w178:dbl, "OK"=w177:bool)  [unwired: 17 in, 1 out]
            n80 = local write "calibrate"(FALSE ("Set Centriod Target")) -> ()
            n81 = case shown="True" w177 {
              tunnel: w180 -> [w184 w191]
              tunnel: [w184 w190] -> w179
              tunnel: w178 -> [_ w186]
              frame False {
              }
              frame True {
                n82 = To Word Integer(number=w186) -> (16bit integer=w185:i16)
                n83 = Number To Decimal String(number=w185) -> (decimal integer string=w187:string)  [unwired: 1 in]
                n84 = call <vilib>:"Build State String with Arguments__jki_lib_state_machine.vi"("Arguments (\"\")"=w187, "State"="Calibrate" ("State(s) at Back (\"\")")) -> ("State with Arguments"=w188:string)  [unwired: 4 in]
                n85 = call <vilib>:"Add State(s) to Queue__jki_lib_state_machine.vi"("State(s) in (\"\")"=w191, "State(s) at Back (\"\")"=w188) -> ("States Out"=w190:string)  [unwired: 13 in]
              }
            }
          }
          event "stop": Value Change {
            # "Exit Button Value Change (pressed) Event\n(this executes Macro: Exit to terminate the VI)"
            n86 = event-data() -> ()  [unwired: 1 in, 6 out]
            n87 = call <vilib>:"Add State(s) to Queue__jki_lib_state_machine.vi"("State(s) in Front (\"\")"="Macro: Exit", "State(s) in (\"\")"=w196) -> ("States Out"=w195:string)  [unwired: 13 in]
          }
          event Panel Close? {
            # "Discard the event because we'll close the front panel ourselves in Macro: Exit"
            # "Close Panel button (pressed) Event\n(this executes Macro: Exit to terminate the VI)"
            n88 = event-data() -> ()  [unwired: 1 in, 1 out]
            n89 = call <vilib>:"Add State(s) to Queue__jki_lib_state_machine.vi"("State(s) in Front (\"\")"="Macro: Exit", "State(s) in (\"\")"=w202) -> ("States Out"=w201:string)  [unwired: 13 in]
            n90 = event-data("Discard?"=TRUE) -> ()  [unwired: 1 in, 1 out]
          }
        }
      }
      frame "---------- Core ----------" {
        # "Do not put any code in this frame.\n(it is a separator no-op)"
        n91 = call <vilib>:"Add State(s) to Queue__jki_lib_state_machine.vi"("State(s) in (\"\")"=w206) -> ("States Out"=w205:string)  [unwired: 14 in]
      }
      frame Default {
        w216 = 42 items=["No error", "Argument error", "Memory is full", "Out of zone", "End of file", "File already open", "Generic file I/O error", "File not found", "File permission error", "Disk is full", "Duplicate path", "Too many files open", "System feature not enabled", "Resource file not found", "Cannot add resource", "Resource not found", "Image not found", "Image memory error", "Pen does not exist", "Config type invalid", "Config token not found", "Config parse error", "Config memory error", "Bad external code format", "Bad external code offset", "External code not present", "Null window", "Destroy window error", "Null menu", "Print aborted", "Bad print record", "Print driver error", "Windows error during printing", "Memory error during printing", "Print dialog error", "Generic print error", "Invalid device refnum", "Device not found", "Device parameter error", "Device unit error", "Cannot open device", "Device call aborted", "Generic error", "Cancelled by user", "Object ID too low", "Object ID too high", "Object not in heap", "Unknown heap", "Unknown object (invalid DefProc)", "Unknown object (DefProc not in table)", "Message out of range", "Invalid (null) method", "Unknown message", "Manager call not supported", "Bad address", "Network operation in progress", "Network operation timed out", "Connection is busy", "Network attribute not supported", "Network error", "Address in use", "System out of memory", "Connection aborted", "Connection refused", "Not connected", "Already connected", "Connection closed", "Initialization error (interapplication manager)", "Bad occurrence", "Wait on unbound occurrence handler", "Occurrence queue overflow", "Datalog type conflict", "Unused", "Unrecognized type (interapplication manager)", "Memory corrupt", "Failed to make temporary DLL", "Old CIN version", "Drag socket not found", "Failed to load drop-object", "Failed to register OLE object", "Failed to release OLE object", "Format specifier type mismatch", "Unknown format specifier", "Too few format specifiers", "Too many format specifiers", "Scan failed", "Newer CIN version", "Error converting to variant", "Runtime menu error", "Password tampered", "Variant attribute not found", "Incompatible variant data type", "Event data is not available", "Event Store is not present", "Occurrence is not found", "Event Queue is not created", "Event info is not available", "Refnum passed is NULL", "Error retrieving Class GUID", "Error retrieving CoClass GUID", "Error retrieving TypeLib GUID.", "Bad built application magic bytes.", "Specific driver is different from the specific driver associated with the Logical Name.", "There is no session opened to the class driver.", "Max Error", "MAX - Error with config objects", "MAX - Error loading configuration", "MAX - Group not supported"]
        # "Current State"
        # "Do not delete, rename, or modify this frame.\n(this is used to capture unhandled states and typos)"
        # "Handle mistyped state name (developer tool)"
        n92 = Format Into String(format string="Software Exception: Unhandled State \"%s\"." ("message"), error in=w212, w207) -> (resulting string=w215:string, error out=w214:errorcluster)  [unwired: 1 in]
        n93 = call <vilib>:"Error Cluster From Error Code.vi"("show call chain? (False)"=TRUE, "error in (no error)"=w214, "error message (\"\")"=w215, "error code (0)"=w216) -> ("error out"=w213:errorcluster)  [unwired: 5 in]
        n94 = call <vilib>:"Add State(s) to Queue__jki_lib_state_machine.vi"("State(s) in (\"\")"=w211) -> ("States Out"=w210:string)  [unwired: 14 in]
      }
      frame "Initialize Core Data" {
        # "Do not delete, rename, or modify this frame.\n(this is used to determine panel behavior on exit)"
        # "originally closed?"
        # "exe?"
        # "If panel starts closed or is an EXE, then close it when we exit"
        n95 = property class="VI"() -> ("Front Panel.Open"=w225:bool)  [unwired: 2 in, 2 out]
        n96 = property class="App"() -> ("App.Kind"=w224:T16)  [unwired: 2 in, 2 out]
        n97 = control-ref of="Current VI Reference"() -> (w218:refnum<vi>)
        n98 = Not(x=w225) -> (.not. x?=w222:bool)
        n99 = Equal?(x=w224, y=T16."Run Time System" ("Application:Kind")) -> (x = y?=w221:bool)
        n100 = Or(x=w222, y=w221) -> (x .or. y?=w219:bool)
        n101 = Bundle By Name(cluster=w220, "Core.Current VI Reference"=w218, "Core.Close Panel on Exit?"=w219) -> (w227:T20)
        n102 = call <vilib>:"Add State(s) to Queue__jki_lib_state_machine.vi"("State(s) in (\"\")"=w229) -> ("States Out"=w228:string)  [unwired: 14 in]
      }
      frame "Error Handler" {
        # "Unhandled Error -- Display it"
        # "Handle any errors here.\nYou can also output any states to clean-up after errors occur"
        # "Clear error"
        n103 = call <vilib>:"General Error Handler.vi"("error in (no error)"=w231) -> ()  [unwired: 10 in, 5 out]
        n104 = call <vilib>:"Add State(s) to Queue__jki_lib_state_machine.vi"("State(s) in Front (\"\")"="/* Post Error States", "State(s) in (\"\")"=w235) -> ("States Out"=w234:string)  [unwired: 13 in]
      }
      frame "Exit" {
        # "Do not put any code in this frame.\n(No errors that occur here will be handled.)"
        n105 = call <vilib>:"Add State(s) to Queue__jki_lib_state_machine.vi"("State(s) in (\"\")"=w240) -> ("States Out"=w239:string)  [unwired: 14 in]
      }
      frame "---------- Data ----------" {
        # "Do not put any code in this frame.\n(It is a separator no-op. You can make a copy of this frame to create a new Data frame)"
        n106 = call <vilib>:"Add State(s) to Queue__jki_lib_state_machine.vi"("State(s) in (\"\")"=w244) -> ("States Out"=w243:string)  [unwired: 14 in]
      }
      frame "Data: Initialize" {
        w250 = T19 {"Slope Axis 1"=0.0, "Axis Inverted"=FALSE, "Slope Axis 2"=0.0, "Axis 1 revered"=FALSE, "Axis 2 revered"=FALSE}  # Motor Calibration
        w251 = FALSE  # set centriod target
        w252 = T1 {"Stat Centriod X"=[], "Stat Centriod Y"=[], "TRA Position X"=[], "TRA PositionY"=[], "Time"=[]}  # Stats
        w254 = FALSE  # moving
        w246 = T5 {"Tolerance [%]"=0.0, "Stepsize"=0.0, "Invert Axis"=FALSE, "Invert Direction X"=FALSE, "Invert Direction Y"=FALSE, "enable feedback"=FALSE, "Set Centriod Target"=FALSE, "my active motor"=""}  # move
        w255 = cluster{"X offset":dbl, "Y offset":dbl} {"X offset"=0.0, "Y offset"=0.0}  # offsets
        w256 = FALSE  # beam detected
        w253 = T3 {"Filter"=1, "Filter Para"={"X Size"=5, "Y Size"=5, "% Tolerance"=1}, "detection method"=4, "smal para"=[{"Measurement Parameter"=35, "Range Lower Value"=0.0, "Range Upper Value"=500.0, "Range"=TRUE, "Measurement Type"=FALSE}], "Remove small Objects"=TRUE, "Restrict to round Objects"=FALSE}  # beam detection para
        w258 = dbl[] []  # Mean Centriod Y
        w259 = dbl[] []  # Mean Centriod X
        w260 = T8 [{"Area"=1104.0, "Number of Holes"=0.0, "Bounding Rect"={"Left"=378.0, "Top"=230.0, "Right"=422.0, "Bottom"=264.0}, "Center of Mass"={"X"=399.60235507246375, "Y"=246.169384057971}, "Orientation"=6.346766143267859, "Dimensions"={"Width"=44.0, "Height"=34.0}}]  # PArticle Report
        w261 = T9 []  # Best Rectangle
        w262 = dbl[] []  # Centriod Y
        w263 = dbl[] []  # Centriod X
        w264 = T22 {"Current VI Reference"=refnum, "Close Panel on Exit?"=FALSE}  # Core
        # "Initialize the shift-register data, here.\n(data names are defined by what you wire into the bundle function)"
        n107 = local read "ActiveMotor"() -> (w248:u16)
        n108 = local write "beam detection para"(w253) -> ()
        n109 = property on="ActiveMotor" class="Ring (strict)"() -> ("Strings []"=w249:string[])  [unwired: 2 in, 2 out]
        n110 = Bundle("Core"=w264, "beam detection para"=w253, "Centriod X"=w263, "Centriod Y"=w262, "Best Rectangle"=w261, "PArticle Report"=w260, "Mean Centriod X"=w259, "Mean Centriod Y"=w258, "Time"="Time", "beam detected"=w256, "offsets"=w255, "move"=w246, "moving"=w254, "Stats"=w252, "set centriod target"=w251, "Motor Calibration"=w250) -> (w266:T20)  [unwired: 1 in]
        n111 = Index Array(array=w249, index=w248) -> (element=w247:string)
        n112 = Bundle By Name(cluster=w246, "my active motor"=w247) -> (w245:T5)
        n113 = property on="ActiveMotorName::2" class="Str"("Val(Sgnl)"=w247) -> ()  [unwired: 2 in, 2 out]
        n114 = call <vilib>:"Add State(s) to Queue__jki_lib_state_machine.vi"("State(s) in (\"\")"=w268) -> ("States Out"=w267:string)  [unwired: 14 in]
        n115 = property on="Move Properties" class="Clust (strict)"("Value"=w245) -> ()  [unwired: 2 in, 2 out]
      }
      frame "Data: Cleanup" {
        # "Cleanup any data and references, here.\n(this is called automatically, by the Macro: Exit)"
        n116 = Unbundle By Name(w270) -> ("Core.Current VI Reference"=w269:refnum<vi>)
        n117 = Close Reference(reference=w269, error in (no error)=w272) -> (error out=w271:errorcluster)
        n118 = call <vilib>:"Add State(s) to Queue__jki_lib_state_machine.vi"("State(s) in (\"\")"=w274) -> ("States Out"=w273:string)  [unwired: 14 in]
      }
      frame "---------- UI ----------" {
        # "Do not put any code in this frame.\n(It is a separator no-op. You can make a copy of this frame to create a new UI frame)"
        n119 = call <vilib>:"Add State(s) to Queue__jki_lib_state_machine.vi"("State(s) in (\"\")"=w278) -> ("States Out"=w277:string)  [unwired: 14 in]
      }
      frame "UI: Initialize" {
        # "Initialize the User Interface, here.\n(this is called automatically, by the Macro: Init)"
        n120 = call <vilib>:"Add State(s) to Queue__jki_lib_state_machine.vi"("State(s) in (\"\")"=w282) -> ("States Out"=w281:string)  [unwired: 14 in]
      }
      frame "UI: Cursor Set" {
        # "Argument"
        # "Set and Unset Cursor Busy.\n(Usage: \"UI: Cursor Set >> Busy|Idle\")"
        n121 = case shown="\"Idle\", Default" w283 {
          tunnel: w285 -> [w290 w292]
          tunnel: [w289 w291] -> w284
          frame "Idle", Default {
            n122 = call <vilib>:"Unset Busy.vi"("error in (no error)"=w290) -> ("error out"=w289:errorcluster)  [unwired: 10 in]
          }
          frame "Busy" {
            n123 = call <vilib>:"Set Busy.vi"("error in (no error)"=w292) -> ("error out"=w291:errorcluster)  [unwired: 9 in, 1 out]
          }
        }
        n124 = call <vilib>:"Add State(s) to Queue__jki_lib_state_machine.vi"("State(s) in (\"\")"=w288) -> ("States Out"=w287:string)  [unwired: 14 in]
      }
      frame "UI: Front Panel State" {
        # "Argument"
        # "Set Front Panel Open or Closed\n(Usage: \"UI: Front Panel State >> Open|Close\")"
        n125 = Unbundle By Name(w295) -> ("Core.Current VI Reference"=w294:refnum<vi>)
        n126 = case shown="\"Close\"" w293 {
          tunnel: w297 -> [w303 w316]
          tunnel: [w305 w317] -> w296
          tunnel: w294 -> [w304 w314]
          frame "Open", Default {
            n127 = property class="VI"(reference=w304, error in=w303) -> (reference out=w301:refnum<vi>, error out=w302:errorcluster, "Front Panel.Open"=w300:bool)
            n128 = case shown="False" w300 {
              tunnel: [w308 w311] -> w305
              tunnel: w302 -> [w307 w311]
              tunnel: w301 -> [w306 _]
              frame False {
                n129 = invoke class="VI" method="FP.Open"(reference=w306, error in=w307, "Activate"=TRUE, "State"=T17."Standard") -> (error out=w308:errorcluster)  [unwired: 1 in, 4 out]
              }
              frame True {
              }
            }
          }
          frame "Close" {
            n130 = property class="VI"(reference=w314, error in=w316) -> (reference out=w313:refnum<vi>, error out=w315:errorcluster, "Front Panel.Open"=w312:bool)
            n131 = case shown="True" w312 {
              tunnel: [w318 w321] -> w317
              tunnel: w315 -> [w318 w320]
              tunnel: w313 -> [_ w319]
              frame False {
              }
              frame True {
                n132 = invoke class="VI" method="FP.Close"(reference=w319, error in=w320) -> (error out=w321:errorcluster)  [unwired: 1 in, 2 out]
              }
            }
          }
        }
        n133 = call <vilib>:"Add State(s) to Queue__jki_lib_state_machine.vi"("State(s) in (\"\")"=w299) -> ("States Out"=w298:string)  [unwired: 14 in]
      }
      frame "---------- Macro ----------" {
        # "Do not put any code in this frame.\n(It is a separator no-op. You can make a copy of this frame to create a new Macro frame)"
        n134 = call <vilib>:"Add State(s) to Queue__jki_lib_state_machine.vi"("State(s) in (\"\")"=w325) -> ("States Out"=w324:string)  [unwired: 14 in]
      }
      frame "Macro: Initialize" {
        w326 = "Data: Initialize\nInitialize Core Data\nUI: Initialize\nUI: Front Panel State >> Open"  # Data: Initialize Initialize Core Data UI: Initialize UI: Front Panel State >> Open
        # "Initialization Macro\n(This is called once, when the VI starts)"
        n135 = call <vilib>:"Add State(s) to Queue__jki_lib_state_machine.vi"("State(s) in Front (\"\")"=w326, "State(s) in (\"\")"=w330) -> ("States Out"=w329:string)  [unwired: 13 in]
      }
      frame "Macro: Exit" {
        # "Exit Macro\n(This is called once, when the VI exits)"
        n136 = Unbundle By Name(w337) -> ("Core.Close Panel on Exit?"=w335:bool)
        n137 = Select(t="UI: Front Panel State >> Close", s=w335, f="") -> (s? t:f=w332:string)
        n138 = call <vilib>:"Add State(s) to Queue__jki_lib_state_machine.vi"("State(s) in (\"\")"=w332, "State(s) at Back (\"\")"="Data: Cleanup\nExit") -> ("States Out"=w336:string)  [unwired: 13 in]
        n139 = call <vilib>:"Add State(s) to Queue__jki_lib_state_machine.vi"("State(s) in Front (\"\")"=w336, "State(s) in (\"\")"=w340) -> ("States Out"=w339:string)  [unwired: 13 in]
      }
      frame "-------------Properties---------" {
        # "Template Separator\n(You can make a copy of, or modify, this frame)"
        n140 = call <vilib>:"Add State(s) to Queue__jki_lib_state_machine.vi"("State(s) in (\"\")"=w344) -> ("States Out"=w343:string)  [unwired: 14 in]
      }
      frame "Beam Detection" {
        # "Your code here.\n(You can make a copy of, or modify, this frame)"
        n141 = Bundle By Name(cluster=w346, "beam detection para"="beam detection para") -> (w345:T20)
        n142 = call <vilib>:"Add State(s) to Queue__jki_lib_state_machine.vi"("State(s) in (\"\")"=w350) -> ("States Out"=w349:string)  [unwired: 14 in]
      }
      frame "Move Properties" {
        n143 = Bundle By Name(cluster=w353, "move"="Move Properties") -> (w352:T20)
        n144 = Unbundle By Name(w352) -> ("move.Stepsize"=w351:dbl)
        n145 = property on="RelativeSettings.Axis 1.StepSize::2" class="DigNum (strict)"("Val(Sgnl)"=w351) -> ()  [unwired: 2 in, 2 out]
        n146 = property on="RelativeSettings.Axis 3.StepSize::2" class="DigNum (strict)"("Val(Sgnl)"=w351) -> ()  [unwired: 2 in, 2 out]
        n147 = call <vilib>:"Add State(s) to Queue__jki_lib_state_machine.vi"("State(s) in (\"\")"=w357) -> ("States Out"=w356:string)  [unwired: 14 in]
      }
      frame "Save Configuration" {
        n148 = Bundle By Name(cluster=w361, "move.enable feedback"=FALSE) -> (w359:T20)
        n149 = local read "GUIdevice 1"() -> (w364:string)
        n150 = local read "ActiveMotor"() -> (w362:u16)
        n151 = local read "GUIdevice 2"() -> (w363:string)
        n152 = local read "stats path"() -> (w358:path)
        n153 = Unbundle By Name(w359) -> ("beam detection para"=w373:T3, "move"=w372:T5)
        n154 = local read "img to avg"() -> (w374:i32)
        n155 = Bundle("img to avg"=w374, "beam detection para"=w373, "move"=w372, "GUIdevice 1"=w364, "GUIdevice 2"=w363, "ActiveMotor"=w362, "stats path"=w358) -> (w371:T6)  [unwired: 1 in]
        n156 = Open/Create/Replace File(error in=w367, operation (0:open)=T18."replace or create with confirmation") -> (refnum out=w375:refnum<file>, error out=w370:errorcluster)  [unwired: 4 in, 1 out]
        n157 = Write to Binary File(file (use dialog)=w375, data=w371, error in=w370) -> (refnum out=w368:refnum<file>, error out=w369:errorcluster)  [unwired: 3 in, 1 out]
        n158 = Close File(refnum=w368, error in=w369) -> (error out=w366:errorcluster)  [unwired: 1 out]
        n159 = local write "Save Config"(FALSE ("Save Button")) -> ()
        n160 = call <vilib>:"Add State(s) to Queue__jki_lib_state_machine.vi"("State(s) in (\"\")"=w378) -> ("States Out"=w377:string)  [unwired: 14 in]
      }
      frame "Save Stats" {
        n161 = local read "Save Stats"() -> (w379:bool)
        n162 = Unbundle By Name(w384) -> ("Stats"=w380:T1)
        n163 = case shown="True" w379 {
          tunnel: w383 -> [w387 w391]
          tunnel: [w387 w390] -> w382
          tunnel: w380 -> [_ w389]
          frame False {
          }
          frame True {
            n164 = Open/Create/Replace File(file path (use dialog)="stats path", error in=w391, operation (0:open)=T18."replace or create") -> (refnum out=w395:refnum<file>, error out=w394:errorcluster)  [unwired: 3 in, 1 out]
            n165 = Write to Binary File(file (use dialog)=w395, data=w389, error in=w394) -> (refnum out=w392:refnum<file>, error out=w393:errorcluster)  [unwired: 3 in, 1 out]
            n166 = Close File(refnum=w392, error in=w393) -> (error out=w390:errorcluster)  [unwired: 1 out]
          }
        }
        n167 = call <vilib>:"Add State(s) to Queue__jki_lib_state_machine.vi"("State(s) in (\"\")"=w386) -> ("States Out"=w385:string)  [unwired: 14 in]
        n168 = local write "Save Stats"(FALSE ("Save Button")) -> ()
      }
      frame "Save Centriod" {
        n169 = local read "Save Stats"() -> (w397:bool)
        n170 = Unbundle By Name(w405) -> ("Time"=w401:timestamp[], "Mean Centriod X"=w400:dbl[], "Mean Centriod Y"=w399:dbl[])
        n171 = Bundle("Time"=w401, "Mean Centriod X"=w400, "Mean Centriod Y"=w399) -> (w398:T2)  [unwired: 1 in]
        n172 = case shown="True" w397 {
          tunnel: w404 -> [w408 w417]
          tunnel: [w408 w416] -> w403
          tunnel: w398 -> [_ w409]
          frame False {
          }
          frame True {
            n173 = local read "stats path"() -> (w415:path)
            n174 = Strip Path(path=w415) -> (stripped path=w411:path, name=w414:string)
            n175 = Concatenate Strings("Centriod_" ("string"), w414) -> (w412:string)
            n176 = Build Path(base path=w411, name or relative path=w412) -> (appended path=w410:path)
            n177 = Open/Create/Replace File(file path (use dialog)=w410, error in=w417, operation (0:open)=T18."replace or create") -> (refnum out=w421:refnum<file>, error out=w420:errorcluster)  [unwired: 3 in, 1 out]
            n178 = Write to Binary File(file (use dialog)=w421, data=w409, error in=w420) -> (refnum out=w418:refnum<file>, error out=w419:errorcluster)  [unwired: 3 in, 1 out]
            n179 = Close File(refnum=w418, error in=w419) -> (error out=w416:errorcluster)  [unwired: 1 out]
          }
        }
        n180 = call <vilib>:"Add State(s) to Queue__jki_lib_state_machine.vi"("State(s) in (\"\")"=w407) -> ("States Out"=w406:string)  [unwired: 14 in]
        n181 = local write "Save Stats"(FALSE ("Save Button")) -> ()
      }
      frame "Load Configuration" {
        # "Your code here.\n(You can make a copy of, or modify, this frame)"
        n182 = Open/Create/Replace File(error in=w433, operation (0:open)=T18."open") -> (refnum out=w440:refnum<file>, error out=w439:errorcluster)  [unwired: 4 in, 1 out]
        n183 = Read from Binary File(5:"output cluster", 8:w439, 11:w440) -> (0:w438:errorcluster, 2:w436:T6, 3:w437:refnum<file>)  [unwired: 3 in, 1 out]
        n184 = Close File(refnum=w437, error in=w438) -> (error out=w432:errorcluster)  [unwired: 1 out]
        n185 = Unbundle By Name(w436) -> ("img to avg"=w425:i32, "beam detection para"=w431:T3, "move"=w430:T5, "GUIdevice 1"=w428:string, "GUIdevice 2"=w427:string, "ActiveMotor"=w424:u16, "stats path"=w423:path)
        n186 = local write "img to avg"(w425) -> ()
        n187 = property on="GUIdevice 2" class="Str"("Val(Sgnl)"=w427) -> ()  [unwired: 2 in, 2 out]
        n188 = local write "ActiveMotor"(w424) -> ()
        n189 = local write "stats path"(w423) -> ()
        n190 = property on="GUIdevice 1" class="Str"("Val(Sgnl)"=w428) -> ()  [unwired: 2 in, 2 out]
        n191 = call <vilib>:"Add State(s) to Queue__jki_lib_state_machine.vi"("State(s) in (\"\")"=w443) -> ("States Out"=w442:string)  [unwired: 14 in]
        n192 = Bundle By Name(cluster=w435, "beam detection para"=w431, "move"=w430) -> (w434:T20)
        n193 = local write "Load Config"(FALSE ("Load Button")) -> ()
        n194 = local write "beam detection para"(w431) -> ()
        n195 = local write "Move Properties"(w430) -> ()
      }
      frame "Reset History" {
        w448 = dbl[] [] ("Mean Centriod X")
        # "Your code here.\n(You can make a copy of, or modify, this frame)"
        n196 = local write "Reset History"(FALSE ("Reset History")) -> ()
        n197 = call <vilib>:"Add State(s) to Queue__jki_lib_state_machine.vi"("State(s) in (\"\")"=w451) -> ("States Out"=w450:string)  [unwired: 14 in]
        n198 = Bundle By Name(cluster=w447, "Mean Centriod X"=w448, "Mean Centriod Y"=w448, "Stats"=T1 {"Stat Centriod X"=[], "Stat Centriod Y"=[], "TRA Position X"=[], "TRA PositionY"=[], "Time"=[]}) -> (w446:T20)
      }
      frame "---------- centriod analysis----------" {
        # "Template Separator\n(You can make a copy of, or modify, this frame)"
        n199 = call <vilib>:"Add State(s) to Queue__jki_lib_state_machine.vi"("State(s) in (\"\")"=w455) -> ("States Out"=w454:string)  [unwired: 14 in]
      }
      frame "detected" {
        w461 = 101 ("y")
        w486 = dbl[] [] ("Array")
        n200 = Unbundle By Name(w471) -> ("Time"=w479:timestamp[], "Centriod X"=w474:dbl[], "Mean Centriod X"=w478:dbl[], "Centriod Y"=w473:dbl[], "Mean Centriod Y"=w477:dbl[], "Best Rectangle"=→"Best Rectangle":T9)
        n201 = local read "Target.X::1"() -> (w476:dbl)
        n202 = local read "Target.Y::1"() -> (w475:dbl)
        n203 = call <vilib>:"Std Deviation and Variance.vi"("X"=w474) -> ("mean"=w480:dbl)  [unwired: 1 in, 2 out]
        "mean X" <- w480
        n204 = call <vilib>:"Std Deviation and Variance.vi"("X"=w473) -> ("mean"=w481:dbl)  [unwired: 1 in, 2 out]
        "mean Y" <- w481
        n205 = Subtract(x=w476, y=w480) -> (x-y=w469:dbl)
        "X offset" <- w469
        n206 = Subtract(x=w475, y=w481) -> (x-y=w468:dbl)
        "Y offset" <- w468
        n207 = Get Date/Time In Seconds() -> (seconds since 1Jan1904=w482:timestamp)
        n208 = Build Array (concatenate)(w478, w469) -> (w458:dbl[])
        n209 = Build Array (concatenate)(w477, w468) -> (w459:dbl[])
        n210 = Build Array (concatenate)(w479, w482) -> (w472:timestamp[])
        n211 = Bundle(w469, w468) -> (w467:cluster{dbl, dbl})  [unwired: 1 in]
        n212 = Array Size(array=w458) -> (size(s)=w463:i32)
        n213 = call <vilib>:"Add State(s) to Queue__jki_lib_state_machine.vi"("State(s) in (\"\")"=w488, "State(s) at Back (\"\")"="check move") -> ("States Out"=w457:string)  [unwired: 13 in]
        n214 = Decrement(x=w461) -> (x-1=w460:i32)
        n215 = Quotient & Remainder(x=w463, y=w461) -> (x-y*floor(x/y)=w462:i32)  [unwired: 1 out]
        n216 = Bundle(w472, w458) -> (w483:cluster{timestamp[], dbl[]})  [unwired: 1 in]
        n217 = Bundle(w472, w459) -> (w484:cluster{timestamp[], dbl[]})  [unwired: 1 in]
        n218 = Equal?(x=w462, y=w460) -> (x = y?=w464:bool)
        n219 = Build Array(w483, w484) -> (→"XY Graph":cluster{timestamp[], dbl[]}[])
        n220 = case shown="True" w464 {
          tunnel: [w489 w491] -> w456
          tunnel: w457 -> [w489 w490]
          frame False {
          }
          frame True {
            n221 = call <vilib>:"Add State(s) to Queue__jki_lib_state_machine.vi"("State(s) in Front (\"\")"=w490, "State(s) at Back (\"\")"="Save Centriod" ("State(s) at Back (\"\")")) -> ("States Out"=w491:string)  [unwired: 13 in]
          }
        }
        n222 = Bundle By Name(cluster=w471, "Time"=w472, "Mean Centriod X"=w458, "Mean Centriod Y"=w459, "Centriod X"=w486, "Centriod Y"=w486, "offsets"=w467) -> (w470:T20)
      }
      frame "check move" {
        n223 = Unbundle By Name(w500) -> ("Best Rectangle"=w518:T9, "offsets.X offset"=w517:dbl, "offsets.Y offset"=w516:dbl)
        n224 = Absolute Value(x=w517) -> (abs(x)=w513:dbl)
        n225 = Absolute Value(x=w516) -> (abs(x)=w510:dbl)
        n226 = Unbundle By Name(w500) -> ("move.Tolerance [%]"=w515:dbl)
        n227 = call "Beam Size.vi"("Best Rectangle"=w518) -> ("Y Size"=w496:dbl, "X Size"=w497:dbl)  [unwired: 9 in]
        "X Size" <- w497
        "Y Size" <- w496
        n228 = Divide(x=w515, y=100.0) -> (x/y=w511:dbl)
        n229 = Max & Min(x=w497, y=w496) -> (max(x,y)=w495:dbl)  [unwired: 1 out]
        n230 = Multiply(x=w511, y=w497) -> (x*y=w512:dbl)
        n231 = Multiply(x=w511, y=w496) -> (x*y=w509:dbl)
        n232 = Divide(x=w495, y=2.0) -> (x/y=w493:dbl)
        n233 = local write "size"(w493) -> ()
        n234 = Greater Or Equal?(x=w513, y=w512) -> (x >= y?=w503:bool)
        n235 = Greater Or Equal?(x=w510, y=w509) -> (x >= y?=w502:bool)
        n236 = Unbundle By Name(w500) -> ("move.enable feedback"=w499:bool)
        n237 = case shown="True" w502 {
          tunnel: w498 -> [w524 w527]
          tunnel: [w524 w525] -> w508
          frame False {
          }
          frame True {
            n238 = call <vilib>:"Add State(s) to Queue__jki_lib_state_machine.vi"("State(s) in (\"\")"=w527, "State(s) at Back (\"\")"="Move Y" ("State(s) at Back (\"\")")) -> ("States Out"=w525:string)  [unwired: 13 in]
          }
        }
        n239 = case shown="True" w503 {
          tunnel: w498 -> [w528 w531]
          tunnel: [w528 w529] -> w507
          frame False {
          }
          frame True {
            n240 = call <vilib>:"Add State(s) to Queue__jki_lib_state_machine.vi"("State(s) in (\"\")"=w531, "State(s) at Back (\"\")"="Move X" ("State(s) at Back (\"\")")) -> ("States Out"=w529:string)  [unwired: 13 in]
          }
        }
        n241 = Or(x=w503, y=w502) -> (x .or. y?=w501:bool)
        n242 = local write "move required"(w501) -> ()
        n243 = Bundle By Name(cluster=w500, "Best Rectangle"=T9 []) -> (w504:T20)
        n244 = case shown="True" w499 {
          tunnel: w508 -> [_ w523]
          tunnel: w507 -> [_ w522]
          tunnel: [w520 w521] -> w506
          tunnel: w498 -> [w520 _]
          frame False {
          }
          frame True {
            n245 = call <vilib>:"Add State(s) to Queue__jki_lib_state_machine.vi"("State(s) in (\"\")"=w522, "State(s) at Back (\"\")"=w523) -> ("States Out"=w521:string)  [unwired: 13 in]
          }
        }
      }
      frame "-----------Motor Move---------" {
        # "Your code here.\n(You can make a copy of, or modify, this frame)"
        n246 = call <vilib>:"Add State(s) to Queue__jki_lib_state_machine.vi"("State(s) in (\"\")"=w535) -> ("States Out"=w534:string)  [unwired: 14 in]
      }
      frame "Move X" {
        w555 = TRUE ("moving")
        n247 = Unbundle By Name(w551) -> ("RelativeMove.Axis 1.CW::2"=w550:refnum<vi>, "RelativeMove.Axis 1.CCW::2"=w549:refnum<vi>, "RelativeMove.Axis 3.CW::2"=w548:refnum<vi>, "RelativeMove.Axis 3.CCW::2"=w547:refnum<vi>)
        n248 = Unbundle By Name(w546) -> ("move.Invert Direction X"=w552:bool, "move.Invert Axis"=w553:bool, "offsets.X offset"=w554:dbl)
        n249 = Greater Than 0?(x=w554) -> (x > 0?=w544:bool)
        n250 = Unbundle By Name(w546) -> ("move.my active motor"=w545:string)
        n251 = stacked-sequence {
          tunnel: w544 -> [_ w567]
          tunnel: w553 -> [_ w566]
          tunnel: w552 -> [_ w565]
          tunnel: w550 -> [_ w564]
          tunnel: w549 -> [_ w563]
          tunnel: w548 -> [_ w562]
          tunnel: w547 -> [_ w561]
          tunnel: w545 -> [w560 _]
          frame #0 {
            n252 = property on="ActiveMotorName::2" class="Str"("Val(Sgnl)"=w560) -> ()  [unwired: 2 in, 2 out]
          }
          frame #1 {
            n253 = case shown="False" w567 {
              tunnel: w566 -> [w573 w593]
              tunnel: w565 -> [w572 w592]
              tunnel: w564 -> [w571 w590]
              tunnel: w563 -> [w570 w591]
              tunnel: w562 -> [w569 w589]
              tunnel: w561 -> [w568 w588]
              frame True {
                n254 = case shown="False" w573 {
                  tunnel: w572 -> [w576 w583]
                  tunnel: w571 -> [w575 _]
                  tunnel: w570 -> [w574 _]
                  tunnel: w569 -> [_ w582]
                  tunnel: w568 -> [_ w581]
                  frame False {
                    n255 = case shown="False" w576 {
                      tunnel: w575 -> [w578 _]
                      tunnel: w574 -> [_ w579]
                      frame False {
                        n256 = property class="Bool (strict)"(reference=w578, "Val(Sgnl)"=TRUE ("Value (Signaling)")) -> ()  [unwired: 1 in, 2 out]
                      }
                      frame True {
                        n257 = property class="Bool (strict)"(reference=w579, "Val(Sgnl)"=TRUE ("Value (Signaling)")) -> ()  [unwired: 1 in, 2 out]
                      }
                    }
                  }
                  frame True {
                    n258 = case shown="False" w583 {
                      tunnel: w582 -> [w584 _]
                      tunnel: w581 -> [_ w586]
                      frame False {
                        n259 = property class="Bool (strict)"(reference=w584, "Val(Sgnl)"=TRUE ("Value (Signaling)")) -> ()  [unwired: 1 in, 2 out]
                      }
                      frame True {
                        n260 = property class="Bool (strict)"(reference=w586, "Val(Sgnl)"=TRUE ("Value (Signaling)")) -> ()  [unwired: 1 in, 2 out]
                      }
                    }
                  }
                }
              }
              frame False {
                n261 = case shown="False" w593 {
                  tunnel: w592 -> [w596 w603]
                  tunnel: w591 -> [w595 _]
                  tunnel: w590 -> [w594 _]
                  tunnel: w589 -> [_ w602]
                  tunnel: w588 -> [_ w601]
                  frame False {
                    n262 = case shown="False" w596 {
                      tunnel: w595 -> [w597 _]
                      tunnel: w594 -> [_ w599]
                      frame False {
                        n263 = property class="Bool (strict)"(reference=w597, "Val(Sgnl)"=TRUE ("Value (Signaling)")) -> ()  [unwired: 1 in, 2 out]
                      }
                      frame True {
                        n264 = property class="Bool (strict)"(reference=w599, "Val(Sgnl)"=TRUE ("Value (Signaling)")) -> ()  [unwired: 1 in, 2 out]
                      }
                    }
                  }
                  frame True {
                    n265 = case shown="True" w603 {
                      tunnel: w602 -> [w604 _]
                      tunnel: w601 -> [_ w606]
                      frame False {
                        n266 = property class="Bool (strict)"(reference=w604, "Val(Sgnl)"=TRUE ("Value (Signaling)")) -> ()  [unwired: 1 in, 2 out]
                      }
                      frame True {
                        n267 = property class="Bool (strict)"(reference=w606, "Val(Sgnl)"=TRUE ("Value (Signaling)")) -> ()  [unwired: 1 in, 2 out]
                      }
                    }
                  }
                }
              }
            }
          }
        }
        n268 = Select(t="pos", s=w544, f="neg") -> (s? t:f=w541:string)
        n269 = Concatenate Strings("x" ("string"), w541) -> (w539:string)
        n270 = call <vilib>:"Build State String with Arguments__jki_lib_state_machine.vi"("Arguments (\"\")"=w539, "State"="Stats") -> ("State with Arguments"=w537:string)  [unwired: 4 in]
        n271 = call <vilib>:"Add State(s) to Queue__jki_lib_state_machine.vi"("State(s) in Front (\"\")"="Wait", "State(s) in (\"\")"=w559, "State(s) at Back (\"\")"=w537) -> ("States Out"=w558:string)  [unwired: 12 in]
        n272 = Bundle By Name(cluster=w546, "moving"=w555) -> (w556:T20)
        n273 = local write "moving"(w555) -> ()
      }
      frame "Move Y" {
        w627 = TRUE ("moving")
        n274 = Unbundle By Name(w623) -> ("RelativeMove.Axis 3.CW::2"=w622:refnum<vi>, "RelativeMove.Axis 3.CCW::2"=w621:refnum<vi>, "RelativeMove.Axis 1.CW::2"=w620:refnum<vi>, "RelativeMove.Axis 1.CCW::2"=w619:refnum<vi>)
        n275 = Unbundle By Name(w618) -> ("move.Invert Direction Y"=w624:bool, "move.Invert Axis"=w625:bool, "offsets.Y offset"=w626:dbl)
        n276 = Greater Than 0?(x=w626) -> (x > 0?=w612:bool)
        n277 = Unbundle By Name(w618) -> ("move.my active motor"=w617:string)
        n278 = stacked-sequence {
          tunnel: w612 -> [_ w639]
          tunnel: w625 -> [_ w638]
          tunnel: w624 -> [_ w637]
          tunnel: w622 -> [_ w636]
          tunnel: w621 -> [_ w635]
          tunnel: w620 -> [_ w634]
          tunnel: w619 -> [_ w633]
          tunnel: w617 -> [w632 _]
          frame #0 {
            n279 = property on="ActiveMotorName::2" class="Str"("Val(Sgnl)"=w632) -> ()  [unwired: 2 in, 2 out]
          }
          frame #1 {
            n280 = case shown="False" w639 {
              tunnel: w638 -> [w645 w665]
              tunnel: w637 -> [w644 w664]
              tunnel: w636 -> [w643 w662]
              tunnel: w635 -> [w642 w663]
              tunnel: w634 -> [w641 w661]
              tunnel: w633 -> [w640 w660]
              frame True {
                n281 = case shown="True" w645 {
                  tunnel: w644 -> [w648 w655]
                  tunnel: w643 -> [w647 _]
                  tunnel: w642 -> [w646 _]
                  tunnel: w641 -> [_ w654]
                  tunnel: w640 -> [_ w653]
                  frame False {
                    n282 = case shown="False" w648 {
                      tunnel: w647 -> [w650 _]
                      tunnel: w646 -> [_ w651]
                      frame False {
                        n283 = property class="Bool (strict)"(reference=w650, "Val(Sgnl)"=TRUE ("Value (Signaling)")) -> ()  [unwired: 1 in, 2 out]
                      }
                      frame True {
                        n284 = property class="Bool (strict)"(reference=w651, "Val(Sgnl)"=TRUE ("Value (Signaling)")) -> ()  [unwired: 1 in, 2 out]
                      }
                    }
                  }
                  frame True {
                    n285 = case shown="True" w655 {
                      tunnel: w654 -> [w656 _]
                      tunnel: w653 -> [_ w658]
                      frame False {
                        n286 = property class="Bool (strict)"(reference=w656, "Val(Sgnl)"=TRUE ("Value (Signaling)")) -> ()  [unwired: 1 in, 2 out]
                      }
                      frame True {
                        n287 = property class="Bool (strict)"(reference=w658, "Val(Sgnl)"=TRUE ("Value (Signaling)")) -> ()  [unwired: 1 in, 2 out]
                      }
                    }
                  }
                }
              }
              frame False {
                n288 = case shown="False" w665 {
                  tunnel: w664 -> [w668 w675]
                  tunnel: w663 -> [w667 _]
                  tunnel: w662 -> [w666 _]
                  tunnel: w661 -> [_ w674]
                  tunnel: w660 -> [_ w673]
                  frame False {
                    n289 = case shown="False" w668 {
                      tunnel: w667 -> [w669 _]
                      tunnel: w666 -> [_ w671]
                      frame False {
                        n290 = property class="Bool (strict)"(reference=w669, "Val(Sgnl)"=TRUE ("Value (Signaling)")) -> ()  [unwired: 1 in, 2 out]
                      }
                      frame True {
                        n291 = property class="Bool (strict)"(reference=w671, "Val(Sgnl)"=TRUE ("Value (Signaling)")) -> ()  [unwired: 1 in, 2 out]
                      }
                    }
                  }
                  frame True {
                    n292 = case shown="True" w675 {
                      tunnel: w674 -> [w676 _]
                      tunnel: w673 -> [_ w678]
                      frame False {
                        n293 = property class="Bool (strict)"(reference=w676, "Val(Sgnl)"=TRUE ("Value (Signaling)")) -> ()  [unwired: 1 in, 2 out]
                      }
                      frame True {
                        n294 = property class="Bool (strict)"(reference=w678, "Val(Sgnl)"=TRUE ("Value (Signaling)")) -> ()  [unwired: 1 in, 2 out]
                      }
                    }
                  }
                }
              }
            }
          }
        }
        n295 = Select(t="pos", s=w612, f="neg") -> (s? t:f=w614:string)
        n296 = Concatenate Strings("y" ("string"), w614) -> (w610:string)
        n297 = call <vilib>:"Build State String with Arguments__jki_lib_state_machine.vi"("Arguments (\"\")"=w610, "State"="Stats") -> ("State with Arguments"=w608:string)  [unwired: 4 in]
        n298 = call <vilib>:"Add State(s) to Queue__jki_lib_state_machine.vi"("State(s) in Front (\"\")"="Wait", "State(s) in (\"\")"=w631, "State(s) at Back (\"\")"=w608) -> ("States Out"=w630:string)  [unwired: 12 in]
        n299 = Bundle By Name(cluster=w618, "moving"=w627) -> (w628:T20)
        n300 = local write "moving"(w627) -> ()
      }
      frame "Wait" {
        w689 = TRUE ("moving")
        # "Wait as long as the motor is moving"
        n301 = Unbundle By Name(w687) -> ("move.Stepsize"=w686:dbl)
        n302 = Multiply(x=w686, y=1.0) -> (x*y=w684:dbl)
        n303 = Add(x=w684, y=100.0) -> (x+y=w682:dbl)
        n304 = call <userlib>:"Wait (ms)__ogtk.vi"("error in (no error)"=w681, "milliseconds to wait"=w682) -> ("error out"=w680:errorcluster)  [unwired: 8 in, 1 out]
        n305 = call <vilib>:"Add State(s) to Queue__jki_lib_state_machine.vi"("State(s) in (\"\")"=w691) -> ("States Out"=w690:string)  [unwired: 14 in]
        n306 = Bundle By Name(cluster=w687, "moving"=w689) -> (w688:T20)
        n307 = local write "moving"(w689) -> ()
      }
      frame "Stats" {
        w699 = 21 ("y")
        # "Your code here.\n(You can make a copy of, or modify, this frame)"
        n308 = Unbundle By Name(w726) -> ("move.Stepsize"=w694:dbl, "Stats.TRA Position X"=w696:dbl[], "Stats.TRA PositionY"=w695:dbl[], "Stats.Stat Centriod X"=w723:dbl[], "Mean Centriod Y"=w722:dbl[], "Stats.Time"=w719:timestamp[])
        n309 = case shown="\"xpos\", Default" w697 {
          tunnel: w696 -> [w734 w742 w751 w759]
          tunnel: w695 -> [w731 w739 w749 w757]
          tunnel: w694 -> [w735 w743 w752 w760]
          tunnel: [w733 w741 w748 w756] -> w692
          tunnel: [w730 w738 w746 w754] -> w693
          frame "xpos", Default {
            n310 = Reverse 1D Array(array=w731) -> (reversed array=w732:dbl[])
            n311 = Reverse 1D Array(array=w734) -> (reversed array=w737:dbl[])
            n312 = Index Array(array=w732) -> (element=w730:dbl)  [unwired: 1 in]
            n313 = Index Array(array=w737) -> (element=w736:dbl)  [unwired: 1 in]
            n314 = Add(x=w736, y=w735) -> (x+y=w733:dbl)
          }
          frame "xneg" {
            n315 = Reverse 1D Array(array=w739) -> (reversed array=w740:dbl[])
            n316 = Reverse 1D Array(array=w742) -> (reversed array=w745:dbl[])
            n317 = Index Array(array=w740) -> (element=w738:dbl)  [unwired: 1 in]
            n318 = Index Array(array=w745) -> (element=w744:dbl)  [unwired: 1 in]
            n319 = Subtract(x=w744, y=w743) -> (x-y=w741:dbl)
          }
          frame "yneg" {
            n320 = Reverse 1D Array(array=w749) -> (reversed array=w750:dbl[])
            n321 = Reverse 1D Array(array=w751) -> (reversed array=w753:dbl[])
            n322 = Index Array(array=w750) -> (element=w747:dbl)  [unwired: 1 in]
            n323 = Index Array(array=w753) -> (element=w748:dbl)  [unwired: 1 in]
            n324 = Subtract(x=w747, y=w752) -> (x-y=w746:dbl)
          }
          frame "ypos" {
            n325 = Reverse 1D Array(array=w757) -> (reversed array=w758:dbl[])
            n326 = Reverse 1D Array(array=w759) -> (reversed array=w761:dbl[])
            n327 = Index Array(array=w758) -> (element=w755:dbl)  [unwired: 1 in]
            n328 = Index Array(array=w761) -> (element=w756:dbl)  [unwired: 1 in]
            n329 = Add(x=w755, y=w760) -> (x+y=w754:dbl)
          }
        }
        n330 = local read "Y offset"() -> (w720:dbl)
        n331 = local read "X offset"() -> (w721:dbl)
        n332 = Get Date/Time In Seconds() -> (seconds since 1Jan1904=w718:timestamp)
        n333 = Decrement(x=w699) -> (x-1=w698:i32)
        n334 = Build Array (concatenate)(w723, w721) -> (w724:dbl[])
        n335 = Build Array (concatenate)(w722, w720) -> (w702:dbl[])
        n336 = Array Size(array=w702) -> (size(s)=w701:i32)
        n337 = Quotient & Remainder(x=w701, y=w699) -> (x-y*floor(x/y)=w700:i32)  [unwired: 1 out]
        n338 = Build Array (concatenate)(w719, w718) -> (w717:timestamp[])
        n339 = Build Array (concatenate)(w696, w692) -> (w727:dbl[])
        n340 = Build Array (concatenate)(w695, w693) -> (w725:dbl[])
        n341 = Equal?(x=w700, y=w698) -> (x = y?=w705:bool)
        n342 = Bundle By Name(cluster=w726, "Stats.TRA Position X"=w727, "Stats.TRA PositionY"=w725, "Stats.Stat Centriod X"=w724, "Stats.Stat Centriod Y"=w702, "Stats.Time"=w717) -> (w716:T20)
        n343 = case shown="True" w705 {
          tunnel: w704 -> [w762 w765]
          tunnel: [w762 w763] -> w703
          frame False {
          }
          frame True {
            n344 = call <vilib>:"Add State(s) to Queue__jki_lib_state_machine.vi"("State(s) in (\"\")"=w765, "State(s) at Back (\"\")"="Save Stats" ("State(s) at Back (\"\")")) -> ("States Out"=w763:string)  [unwired: 13 in]
          }
        }
        n345 = Unbundle By Name(w716) -> ("Stats.Time"=w712:timestamp[], "Stats.Stat Centriod X"=w715:dbl[], "Stats.Stat Centriod Y"=w714:dbl[], "Stats.TRA Position X"=w713:dbl[], "Stats.TRA PositionY"=w711:dbl[])
        n346 = call <vilib>:"Add State(s) to Queue__jki_lib_state_machine.vi"("State(s) in (\"\")"=w703) -> ("States Out"=w729:string)  [unwired: 14 in]
        n347 = Bundle("Time"=w712, "Stat Centriod X"=w715) -> (w710:T23)  [unwired: 1 in]
        n348 = Bundle("Time"=w712, "Stat Centriod Y"=w714) -> (w709:T24)  [unwired: 1 in]
        n349 = Bundle("Time"=w712, "TRA Position X"=w713) -> (w708:T25)  [unwired: 1 in]
        n350 = Bundle("Time"=w712, "TRA PositionY"=w711) -> (w707:T26)  [unwired: 1 in]
        n351 = Build Array(w710, w709, w708, w707) -> (→"Stats":T27)
      }
      frame "Calibrate" {
        # "Your code here.\n(You can make a copy of, or modify, this frame)"
        n352 = Unbundle By Name(w777) -> ("RelativeMove.Axis 1.CW::2"=w770:refnum<vi>, "RelativeMove.Axis 1.CCW::2"=w769:refnum<vi>)
        n353 = control-ref of="RelativeSettings.Axis 1.Position::2"() -> (w768:refnum<vi>)
        n354 = Unbundle By Name(w776) -> ("beam detection para"=w772:T3)
        n355 = Decimal String To Number(string=w774) -> (number=w771:i32)  [unwired: 2 in, 1 out]
        n356 = Build Array(w768, w768) -> (w767:refnum<vi>[])
        n357 = Build Array(w770, w769) -> (w766:refnum<vi>[])
        n358 = call "CalibrateSingleAxis.vi"("Numeric"=w771, "beam detection para"=w772, "error in (no error)"=w775, "RelativeSettings.Axis 1"=w767, "RelativeMove.Axis 1"=w766, "Refnum in"=w773) -> ()  [unwired: 2 in, 4 out]
        n359 = call <vilib>:"Add State(s) to Queue__jki_lib_state_machine.vi"("State(s) in (\"\")"=w779) -> ("States Out"=w778:string)  [unwired: 14 in]
      }
      frame "New Category: 2" {
        # "Your code here.\n(You can make a copy of, or modify, this frame)"
        n360 = call <vilib>:"Add State(s) to Queue__jki_lib_state_machine.vi"("State(s) in (\"\")"=w783) -> ("States Out"=w782:string)  [unwired: 14 in]
      }
    }
    n361 = disable-structure shown="Disabled" {
      disable-tunnel: "ActiveMotorName::2" -> [w54 _]
      disable-tunnel: "ActiveMotor" -> [w51 _]
      frame Disabled {
        n362 = property on="ActiveMotor" class="Ring (strict)"() -> ("Strings []"=w50:string[])  [unwired: 2 in, 2 out]
        n363 = Index Array(array=w50, index=w51) -> (element=w52:string)
        n364 = Not Equal?(x=w54, y=w52) -> (x != y?=w53:bool)
        n365 = case shown="True" w53 {
          tunnel: w50 -> [_ w57]
          tunnel: w54 -> [_ w56]
          frame False {
          }
          frame True {
            n366 = Search 1D Array(1D array=w57, element=w56) -> (index of element=w55:i32)  [unwired: 1 in]
            n367 = property on="ActiveMotor" class="Ring (strict)"("Value"=w55) -> ()  [unwired: 2 in, 2 out]
          }
        }
      }
      frame Enabled {
      }
    }
  }
  n368 = control-ref of="This Application"() -> (w11:refnum<vi>)
  n369 = control-ref of="This VI"() -> (w15:refnum<vi>)
  n370 = Current VI's Menubar() -> (w14:refnum<k9>)
  n371 = call "supergui create stop queue.vi"() -> ("STOP Queue out"=w1:refnum<queue>)  [unwired: 11 in]
  n372 = call "GUI_Master_subvi_reentrant_queues.vi"("STOP Queue in"=w1, "This Application"=w11, "error in (no error)"=w12, "tcp data event"=w10, "Caller menu reference"=w14, "Caller VI ref"=w15) -> ("error out"=w23:errorcluster)  [unwired: 5 in]
  n373 = call <vilib>:"Clear Errors.vi"("error in (no error)"=w23) -> ("error out"=w21:errorcluster)  [unwired: 5 in, 1 out]
  n374 = call "IMAQ Dispose"("error in (no error)"=w21) -> ("error out"=w20:errorcluster)  [unwired: 5 in]
  n375 = call "IMAQ Dispose"("Image"=w16, "error in (no error)"=w20) -> ("error out"=→"error IO 2":errorcluster)  [unwired: 4 in]
